vi "Modbus Message Loop.vi"(0 "Message Queues in":T1, 1 "PLC IP address":string="10.2.0.11", 3 "error in (no error)":errorcluster) -> (10 "error out":errorcluster)   [LabVIEW 2020, in "Modbus.lvlib"]
uses:
  Modbus.lvlib
  support/Message Queue/All Message Queues.ctl
  support/Message Queue/Message Cluster.ctl
  <vilib>/NI/Modbus Library/API/Master/Modbus Master.lvclass
  support/Message Queue/Enqueue Message (Single).vi
  <vilib>/NI/Modbus Library/API/Wrapper/Create TCP Master.vi
  support/Message Queue/Message Queue.lvlib
  <vilib>/NI/Modbus Library/API/Wrapper/API Main.lvlib
panel:
  out "LDO Array 2":bool[](array[boolean])
  in  "Read States":bool
  out "States":string[](array[string])
  out "TimeoutRequestGetDataLDO":u16[](array[numeric])
  out "LDO Array 1":bool[](array[boolean])
  out "Loop Count":i32
  out "FV Output":bool[](array[boolean])
  out "TimeoutRequestGetDataFVIR":i32[](array[numeric])
  out "Input Registers":u16[](array[numeric])
  # "Anybus: 192.168.0.50\nPLC: 192.168.0.20\n\nThis is available in the front HMI, e. IP and port. Useful for debugging and IP config change"
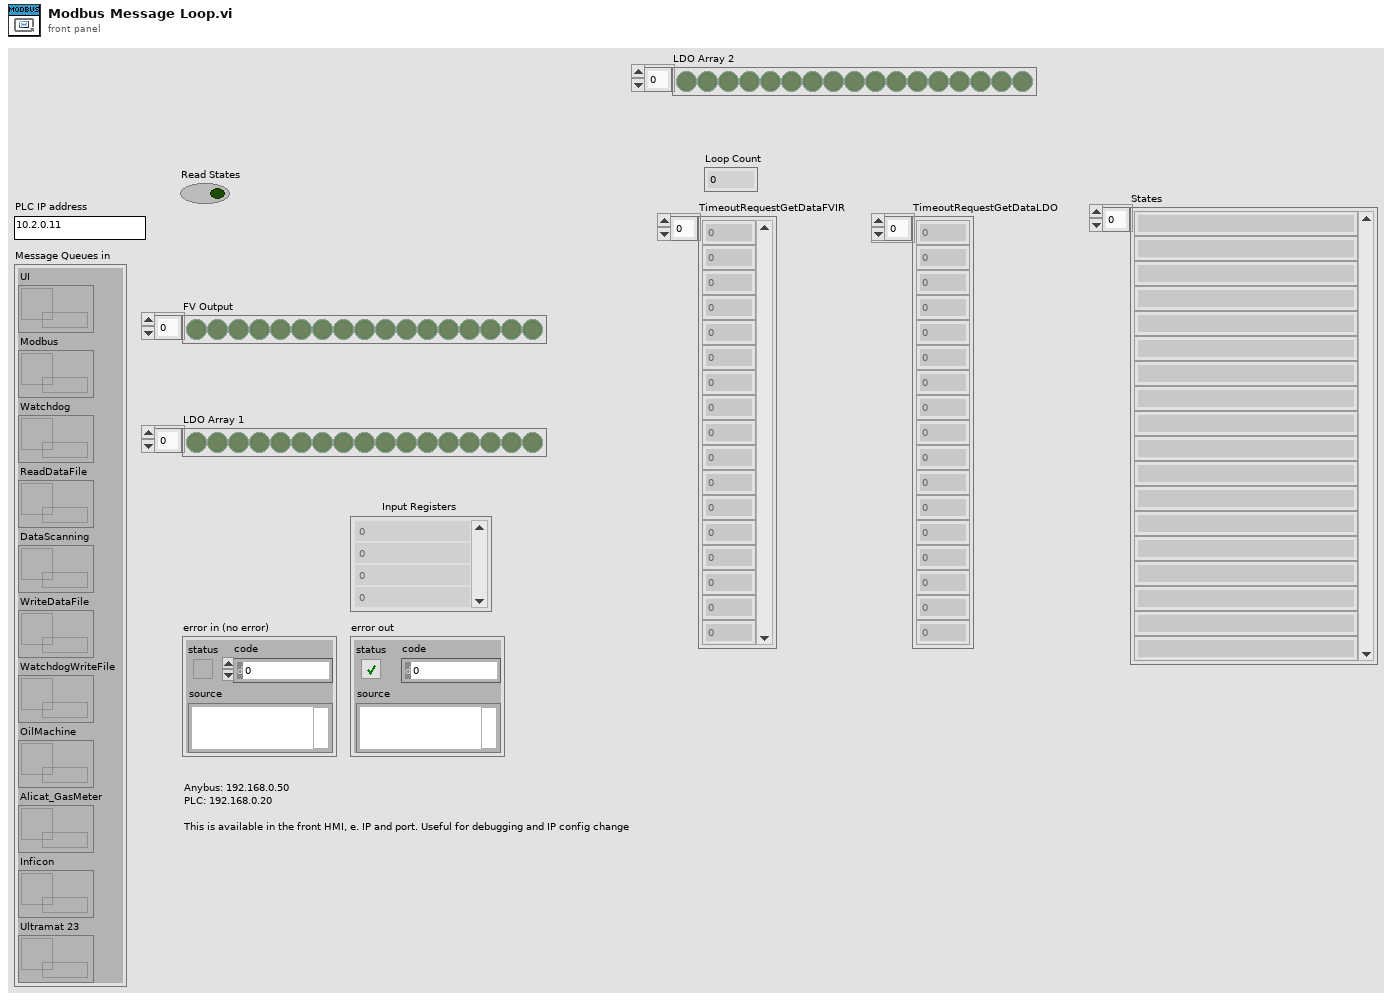
[diagram p1: front panel]
types:
  T1 = typedef "Message Queue.lvlib/All Message Queues.ctl" = cluster{"UI":refnum<queue>, "Modbus":refnum<queue>, "Watchdog":refnum<queue>, "ReadDataFile":refnum<queue>, "DataScanning":refnum<queue>, "WriteDataFile":refnum<queue>, "WatchdogWriteFile":refnum<queue>, "OilMachine":refnum<queue>, "Alicat_GasMeter":refnum<queue>, "Inficon":refnum<queue>, "Ultramat 23":refnum<queue>}
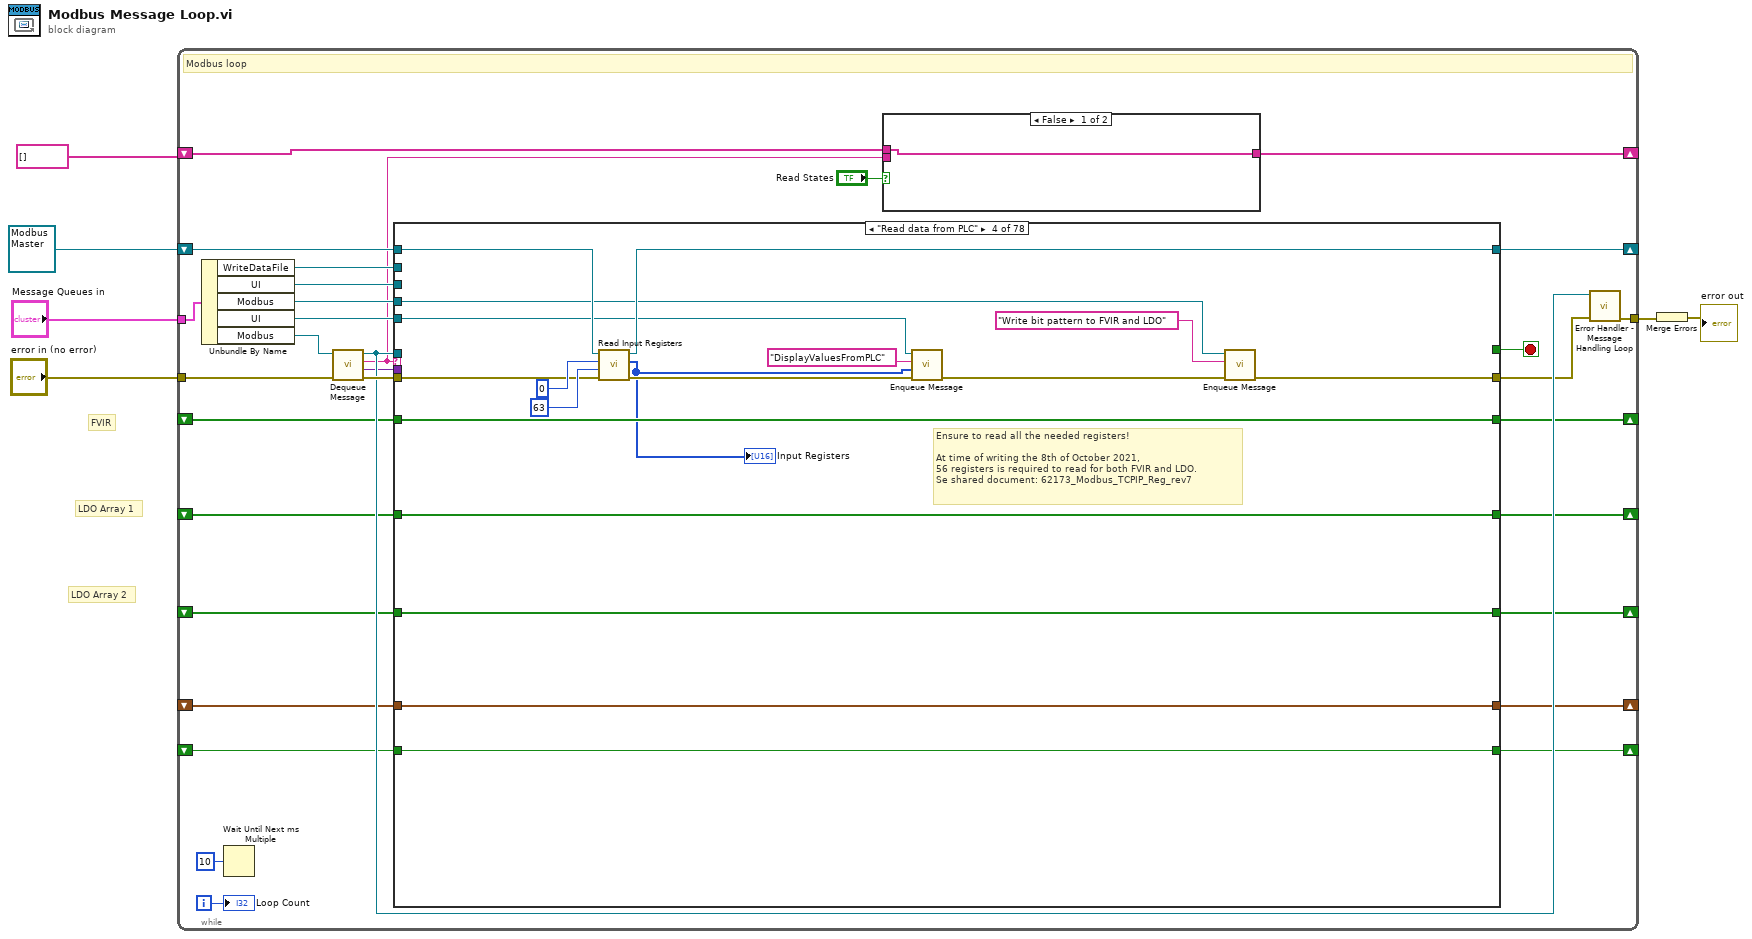
[diagram p0: block diagram]
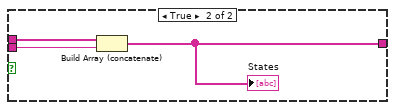
[diagram p2: hidden frame]
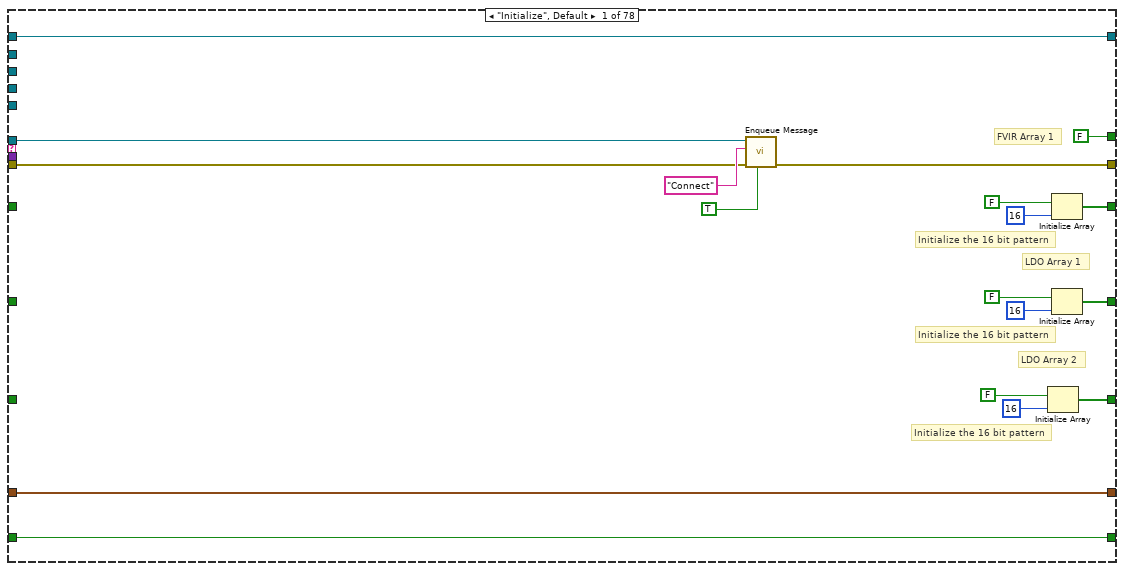
[diagram p3: hidden frame]
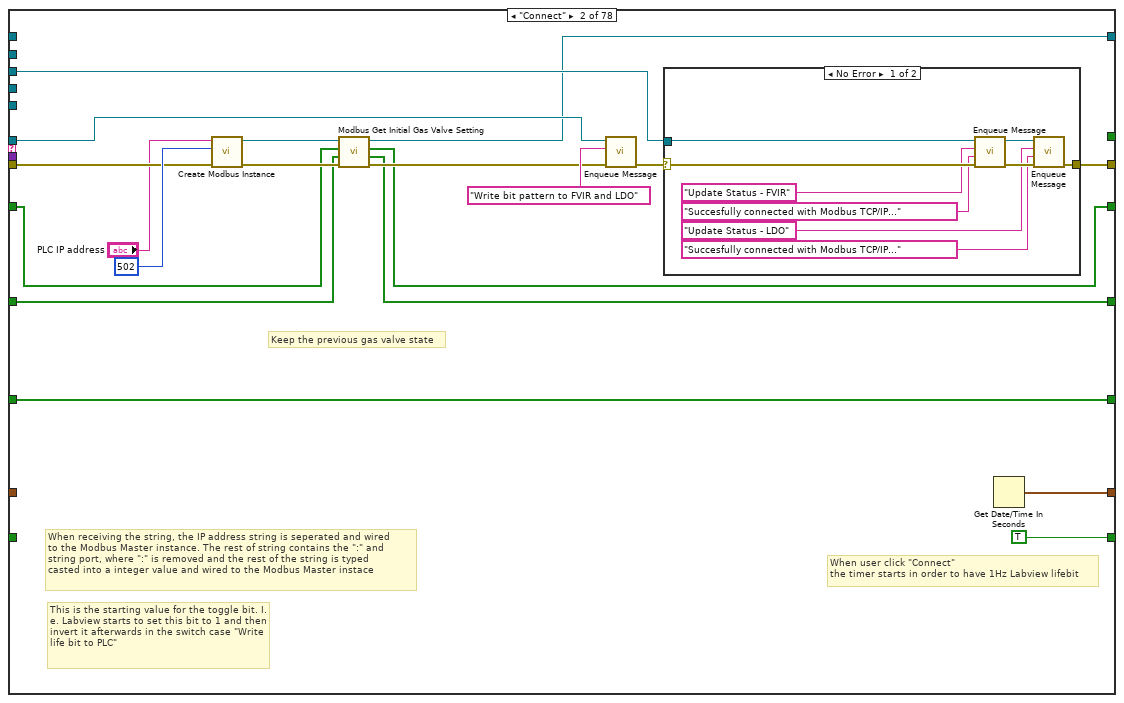
[diagram p4: hidden frame]
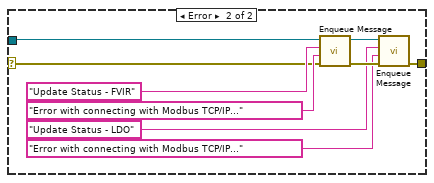
[diagram p5: hidden frame]
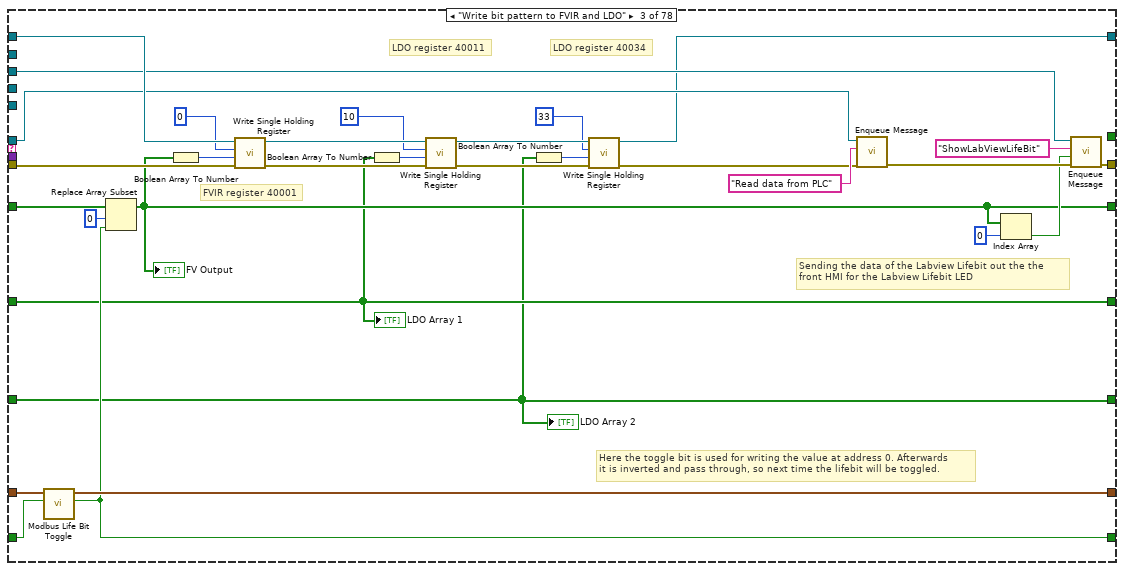
[diagram p6: hidden frame]
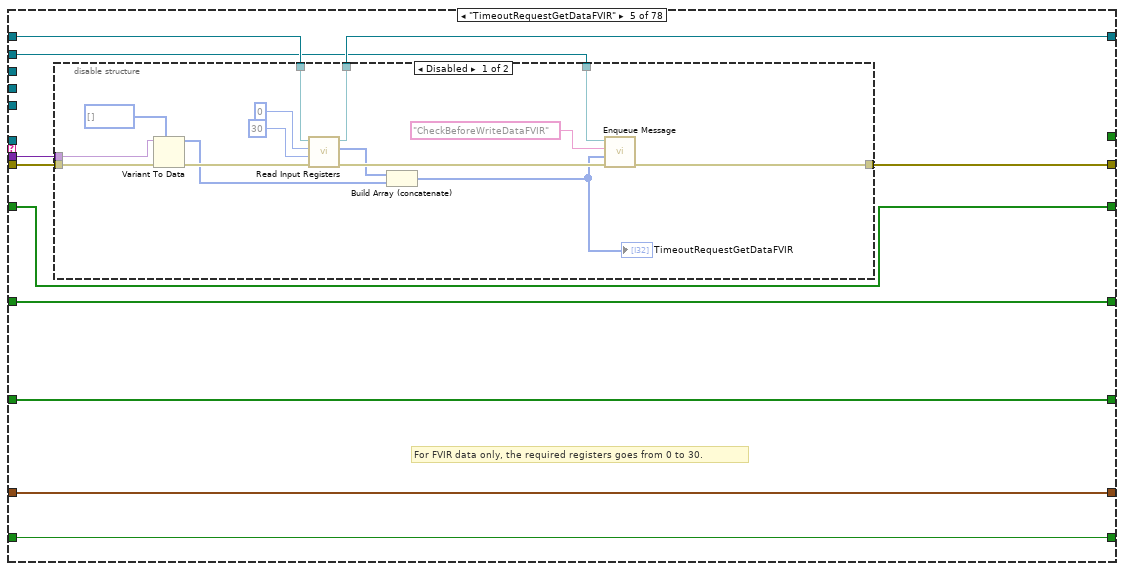
[diagram p7: hidden frame]
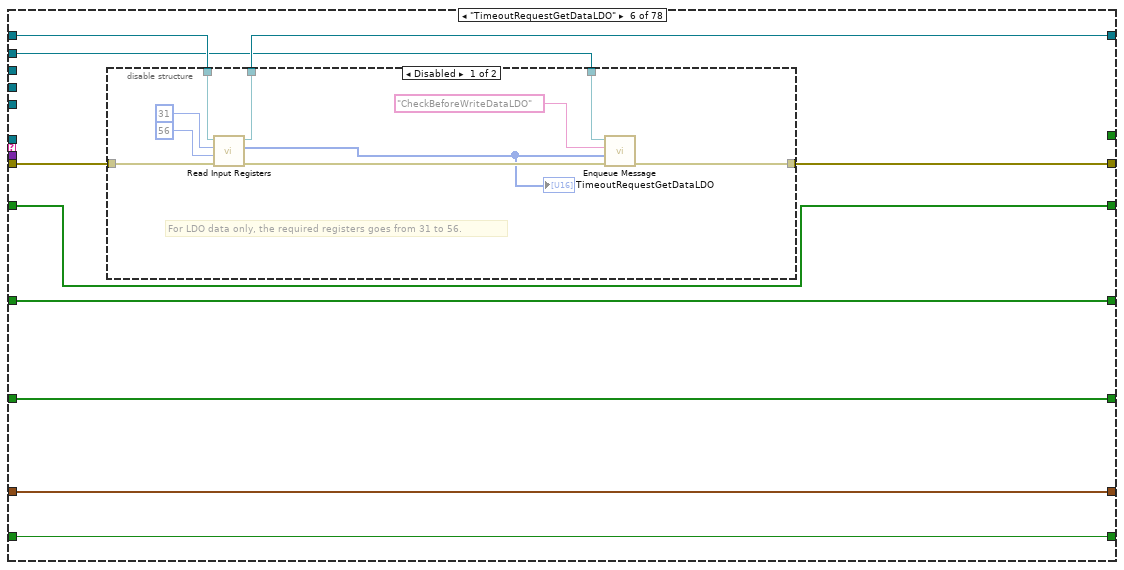
[diagram p9: hidden frame]
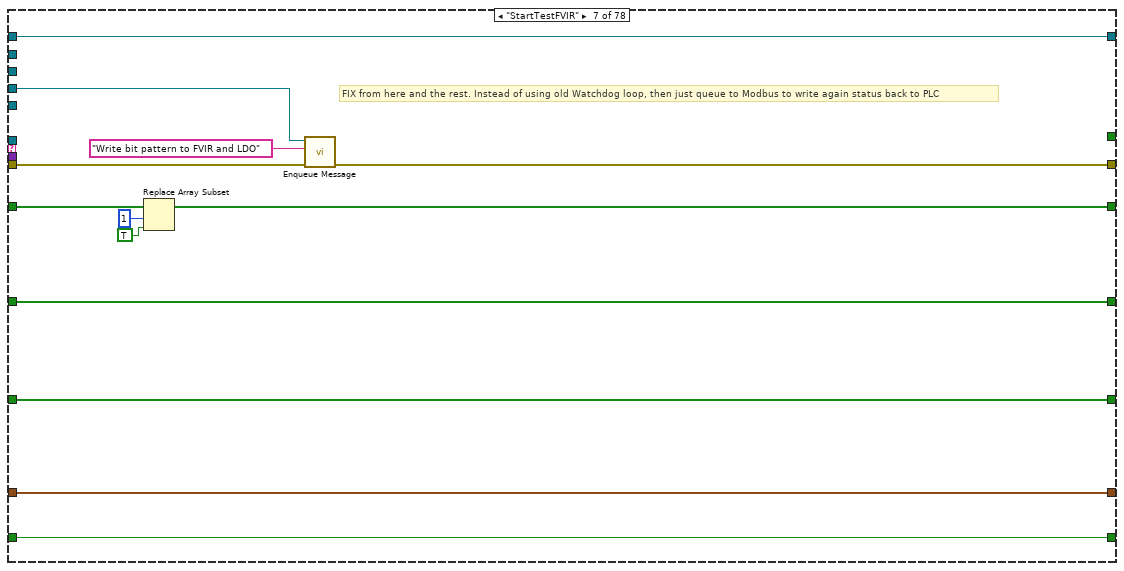
[diagram p11: hidden frame]
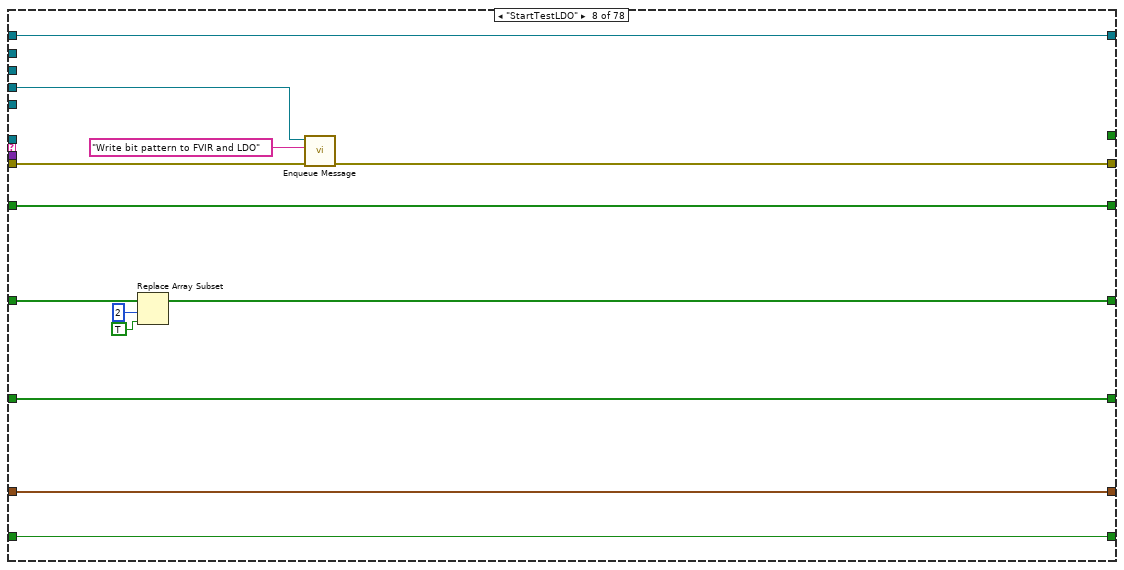
[diagram p12: hidden frame]
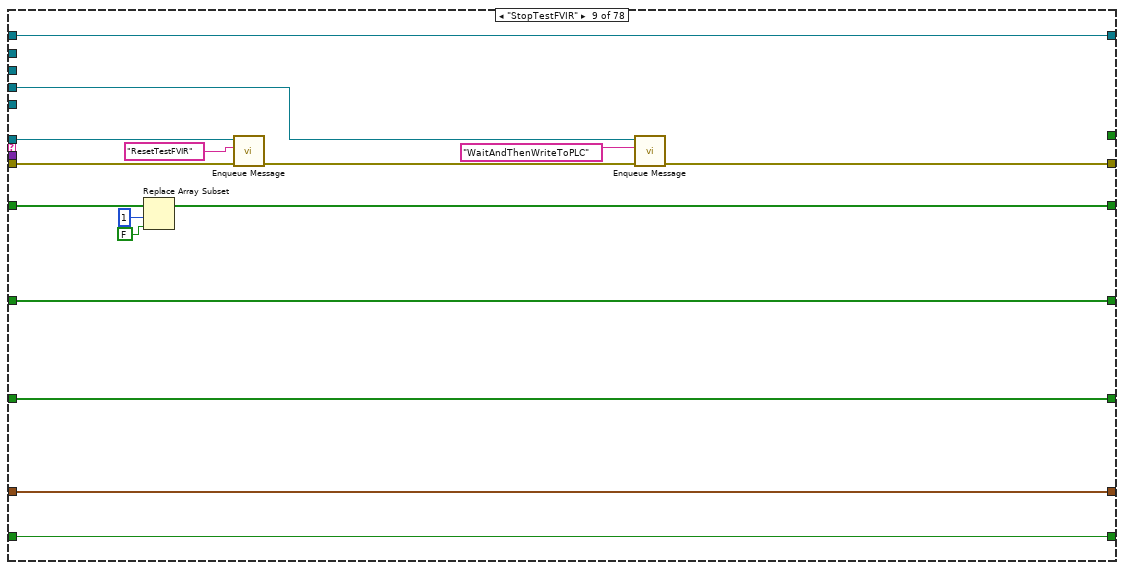
[diagram p13: hidden frame]
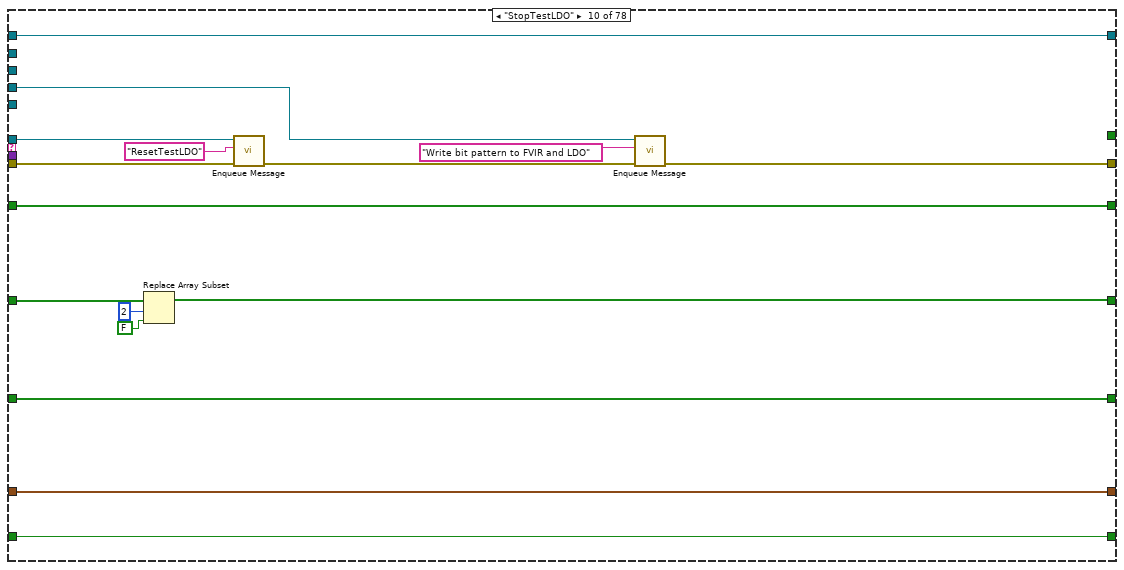
[diagram p14: hidden frame]
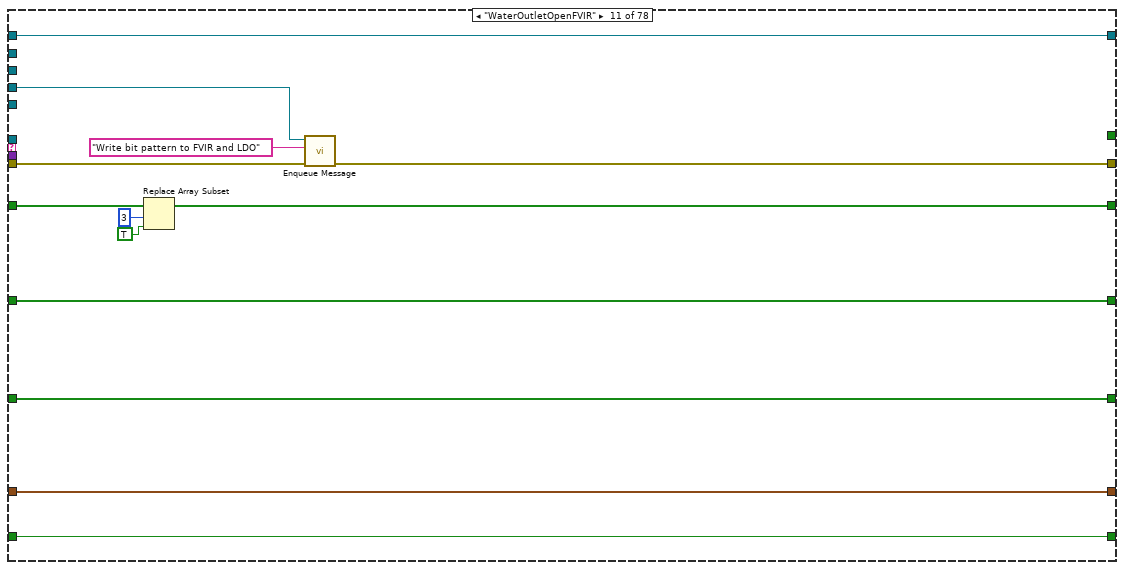
[diagram p15: hidden frame]
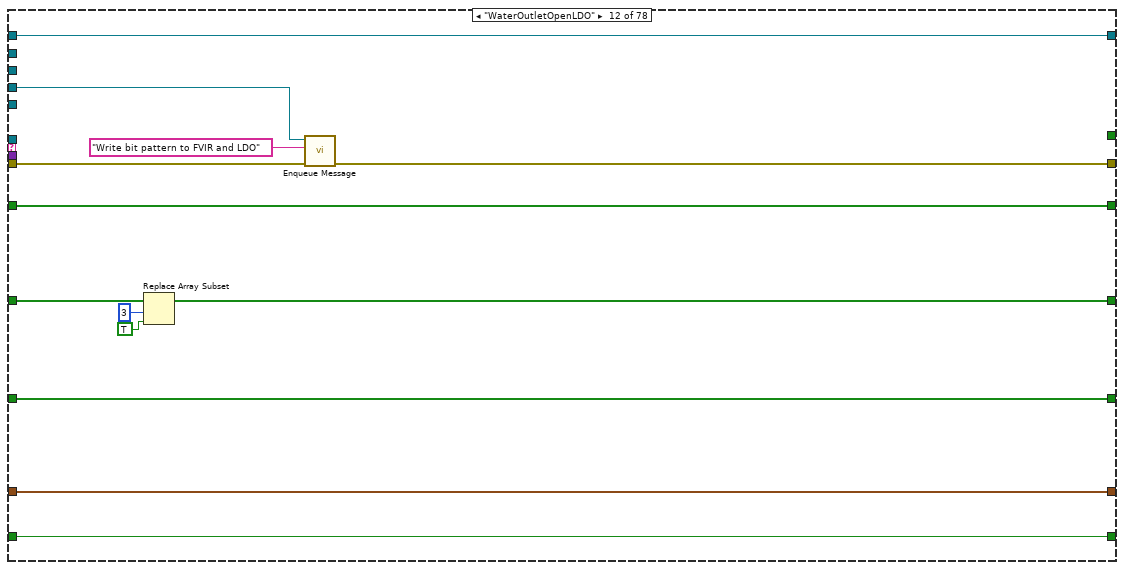
[diagram p16: hidden frame]
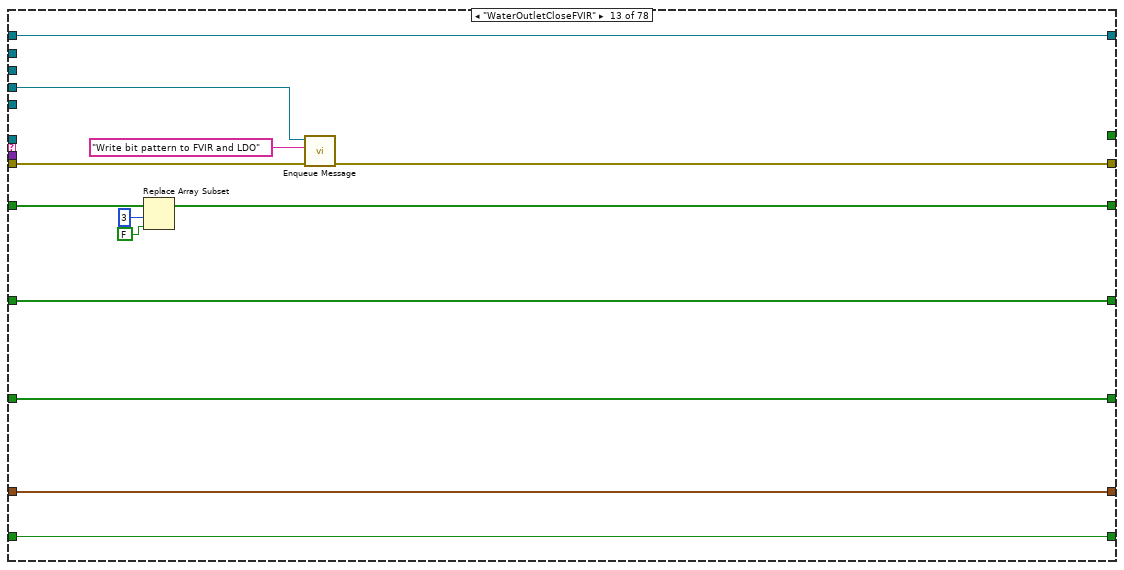
[diagram p17: hidden frame]
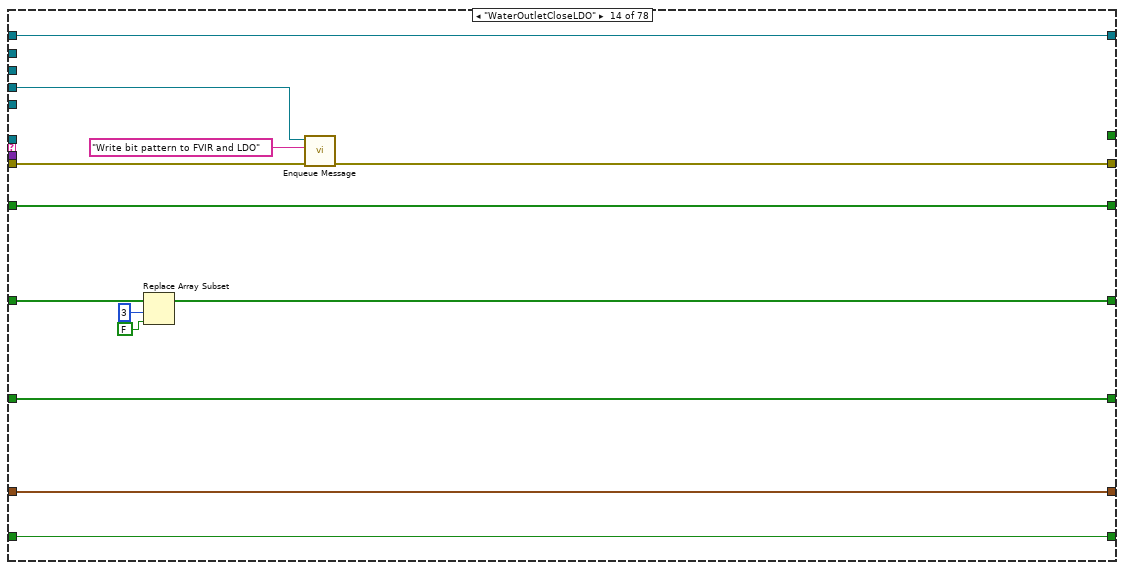
[diagram p18: hidden frame]
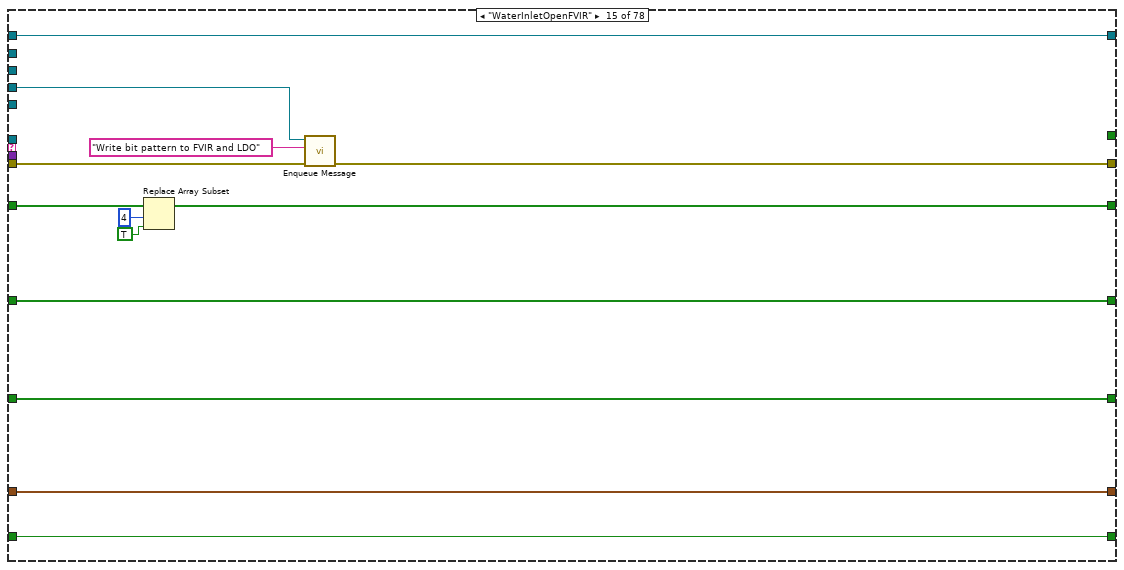
[diagram p19: hidden frame]
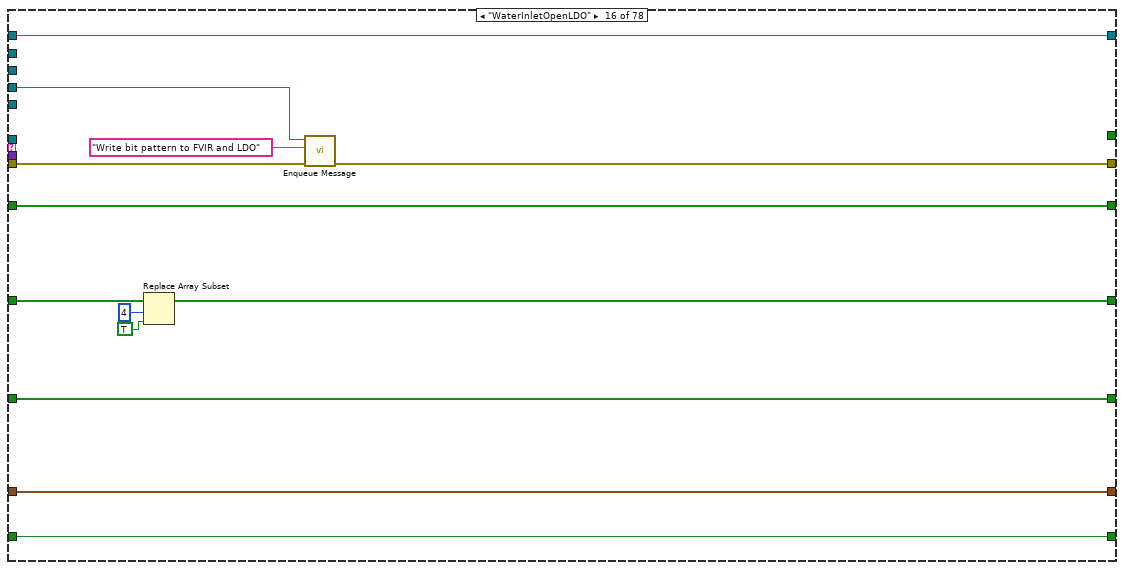
[diagram p20: hidden frame]
diagram:
  # "LDO Array 2"
  # "LDO Array 1"
  # "FVIR"
  n1 = while {
    tunnel: "Message Queues in" -> [w35]
    tunnel: [w34] -> w3
    tunnel: "error in (no error)" -> [w33]
    shift-right: [w31] -> _
    shift-left: refnum<class "Modbus Master.lvclass"> refnum ("Modbus Master") -> [w32]
    shift-right: [w25] -> _
    shift-left: _ -> [w24]
    shift-right: [w21] -> _
    shift-left: _ -> [w20]
    shift-right: [w18] -> _
    shift-left: _ -> [w17]
    shift-right: [w16] -> _
    shift-left: _ -> [w15]
    shift-right: [w10] -> _
    shift-left: string[] [] -> [w12]
    shift-right: [w8] -> _
    shift-left: _ -> [w7]
    i -> [w13]
    stop <- w36 stop-if-true
    # "Modbus loop"
    n2 = Unbundle By Name(w35) -> ("WriteDataFile"=w19:refnum<queue>, "UI"=w23:refnum<queue>, "Modbus"=w29:refnum<queue>, "UI"=w27:refnum<queue>, "Modbus"=w28:refnum<queue>)
    n3 = Wait Until Next ms Multiple(millisecond multiple=u32 10) -> ()  [unwired: 1 out]
    n4 = call "Dequeue Message.vi"("error in (no error)"=w33, "Message Queue"=w28) -> ("error out"=w37:errorcluster, "Message Data"=w26:variant, "Message"=w11:string, "dup Message Queue"=w30:refnum<queue>)  [unwired: 6 in]
    n5 = case shown="\"Read data from PLC\"" w11 {
      tunnel: w30 -> [w46 w74 w113 _ _ _ _ _ w228 w246 _ _ _ _ _ _ _ _ _ _ _ _ _ _ _ _ _ _ _ _ _ _ _ _ _ _ _ _ _ _ _ _ _ _ _ _ _ _ _ _ _ _ _ _ _ _ _ _ _ _ _ _ _ _ _ _ _ _ _ _ _ _ w1127 _ _ _ _ _]
      tunnel: w37 -> [w48 w70 w114 w137 w150 w180 w205 w217 w227 w245 w262 w275 w288 w301 w314 w327 w340 w353 w366 w379 w392 w405 w418 w431 w444 w457 w470 w483 w496 w509 w518 w529 w548 w561 w574 w587 w600 w613 w626 w639 w647 w660 w673 w686 w699 w712 w734 w745 w762 w773 w790 w801 w818 w829 w847 w861 w875 w889 w903 w917 w923 w945 w959 w973 w978 w990 w1004 w1017 _ _ w1076 w1088 w1117 w1159 w1178 w1197 w1211 w1230]
      tunnel: [w47 w77 w123 w132 w152 w178 w207 w220 w230 w248 w265 w278 w291 w304 w317 w330 w343 w356 w369 w382 w395 w408 w421 w434 w447 w460 w473 w486 w499 w512 w515 w528 w551 w564 w577 w590 w603 w616 w629 w642 w646 w659 w672 w685 w698 w711 w728 w748 w756 w776 w784 w804 w812 w832 w839 w853 w867 w881 w895 w909 w924 w937 w951 w965 w979 w992 w1005 w1018 w1037 w1061 w1072 w1081 w1110 w1148 w1166 w1185 w1205 w1224] -> w22
      tunnel: [FALSE _ _ _ _ _ _ _ _ _ _ _ _ _ _ _ _ _ _ _ _ _ _ _ _ _ _ _ _ _ _ _ _ _ _ _ _ _ _ _ _ _ _ _ _ _ _ _ _ _ _ _ _ _ _ _ _ _ _ _ _ _ _ _ _ _ _ _ _ _ _ _ TRUE _ _ _ _ _] -> w36
      tunnel: w32 -> [w59 _ w127 w144 w156 w183 w206 w218 w236 w252 w263 w276 w289 w302 w315 w328 w341 w354 w367 w380 w393 w406 w419 w432 w445 w458 w471 w484 w497 w510 w523 w536 w549 w562 w575 w588 w601 w614 w627 w640 w645 w658 w671 w684 w697 w710 w735 w746 w763 w774 w791 w802 w819 w830 w845 w859 w873 w887 w901 w915 w930 w943 w957 w971 w974 w987 w1000 w1013 w1034 w1059 w1074 w1087 w1113 w1152 w1171 w1190 w1209 w1228]
      tunnel: [w59 w65 w100 w142 w155 w182 w206 w218 w236 w252 w263 w276 w289 w302 w315 w328 w341 w354 w367 w380 w393 w406 w419 w432 w445 w458 w471 w484 w497 w510 w523 w536 w549 w562 w575 w588 w601 w614 w627 w640 w645 w658 w671 w684 w697 w710 w735 w746 w763 w774 w791 w802 w819 w830 w846 w860 w874 w888 w902 w916 w931 w944 w958 w972 w974 w987 w1000 w1013 w1033 w1058 w1075 w1087 w1113 w1151 w1170 w1189 w1208 w1227] -> w31
      tunnel: w29 -> [_ _ _ w131 _ _ w208 w221 w231 w249 w266 w279 w292 w305 w318 w331 w344 w357 w370 w383 w396 w409 w422 w435 w448 w461 w474 w487 w500 w513 w519 w530 w552 w565 w578 w591 w604 w617 w630 w643 w648 w661 w674 w687 w700 w713 w727 w749 w755 w777 w783 w805 w811 w833 w842 w856 w870 w884 w898 w912 w927 w940 w954 w968 w977 w991 w1003 w1016 w1041 w1065 _ w1085 w1116 w1147 w1168 w1187 w1204 w1223]
      tunnel: w27 -> [_ _ _ w140 _ _ _ _ _ _ _ _ _ _ _ _ _ _ _ _ _ _ _ _ _ _ _ _ _ _ _ _ _ _ _ _ _ _ _ _ _ _ _ _ _ _ _ _ _ _ _ _ _ _ _ _ _ _ _ _ _ _ _ _ _ _ _ _ _ _ _ _ w1109 _ _ _ _ _]
      tunnel: w26 -> [_ _ _ _ w149 _ _ _ _ _ _ _ _ _ _ _ _ _ _ _ _ _ _ _ _ _ _ _ _ _ _ _ _ _ _ _ _ _ _ _ _ _ _ _ _ _ _ _ _ _ _ _ _ _ _ _ _ _ _ _ _ _ _ _ _ _ _ _ w1039 w1063 _ _ _ w1158 w1177 w1196 w1210 w1229]
      tunnel: [w55 w63 w107 w138 w154 w181 w202 w212 w233 w243 w259 w270 w285 w296 w311 w322 w337 w348 w363 w374 w389 w400 w415 w426 w441 w452 w467 w478 w493 w504 w526 w539 w543 w556 w569 w582 w595 w608 w621 w634 w656 w669 w682 w695 w708 w721 w731 w742 w759 w770 w787 w798 w815 w826 w838 w852 w866 w880 w894 w908 w922 w936 w950 w964 w986 w999 w1012 w1025 w1030 w1055 w1070 w1084 w1122 w1164 w1183 w1202 w1221 w1240] -> w25
      tunnel: w24 -> [_ w64 w108 w138 w154 w181 w203 w212 w234 w243 w260 w270 w286 w296 w312 w322 w338 w348 w364 w374 w390 w400 w416 w426 w442 w452 w468 w478 w494 w504 w526 w539 w543 w556 w569 w582 w595 w608 w621 w634 w656 w669 w682 w695 w708 w721 w732 w743 w760 w771 w788 w799 w816 w827 w838 w852 w866 w880 w894 w908 w922 w936 w950 w964 w986 w999 w1012 w1025 w1030 w1055 w1070 w1084 w1122 w1164 w1183 w1202 w1221 w1240]
      tunnel: w23 -> [_ w78 w121 _ _ _ _ _ _ _ _ _ _ _ _ _ _ _ _ _ _ _ _ _ _ _ _ _ _ _ _ _ _ _ _ _ _ _ _ _ _ _ _ _ _ _ _ _ _ _ _ _ _ _ _ _ _ _ _ _ _ _ _ _ _ _ _ _ _ _ _ w1080 _ _ _ _ _ _]
      tunnel: [w52 w61 w104 w134 w153 w179 w200 w213 w225 w241 w257 w271 w283 w297 w309 w323 w335 w349 w361 w375 w387 w401 w413 w427 w439 w453 w465 w479 w491 w505 w516 w531 w544 w557 w570 w583 w596 w609 w622 w635 w650 w663 w676 w689 w702 w715 w725 w740 w753 w768 w781 w796 w809 w824 w837 w851 w865 w879 w893 w907 w921 w935 w949 w963 w985 w998 w1011 w1024 w1029 w1054 w1069 w1083 w1121 w1163 w1182 w1201 w1220 w1239] -> w21
      tunnel: w20 -> [_ w62 w104 w134 w153 w179 w200 w214 w225 w242 w257 w272 w283 w298 w309 w324 w335 w350 w361 w376 w387 w402 w413 w428 w439 w454 w465 w480 w491 w506 w517 w532 w545 w558 w571 w584 w597 w610 w623 w636 w651 w664 w677 w690 w703 w716 w725 w740 w753 w768 w781 w796 w809 w824 w837 w851 w865 w879 w893 w907 w921 w935 w949 w963 w985 w998 w1011 w1024 w1029 w1054 w1069 w1083 w1121 w1163 w1182 w1201 w1220 w1239]
      tunnel: w19 -> [_ _ _ _ w151 w177 _ _ _ _ _ _ _ _ _ _ _ _ _ _ _ _ _ _ _ _ _ _ _ _ _ _ _ _ _ _ _ _ _ _ _ _ _ _ _ _ _ _ _ _ _ _ _ _ _ _ _ _ _ _ _ _ _ _ _ _ _ _ _ _ _ _ _ _ _ _ _ _]
      tunnel: [w51 w73 w111 w130 w148 w176 w198 w211 w224 w240 w256 w269 w282 w295 w308 w321 w334 w347 w360 w373 w386 w399 w412 w425 w438 w451 w464 w477 w490 w503 w525 w538 w542 w555 w568 w581 w594 w607 w620 w633 w655 w668 w681 w694 w707 w720 w724 w739 w752 w767 w780 w795 w808 w823 w836 w850 w864 w878 w892 w906 w920 w934 w948 w962 w984 w997 w1010 w1023 w1028 w1053 w1068 w1079 w1120 w1162 w1181 w1200 w1219 w1238] -> w18
      tunnel: w17 -> [w51 _ w110 w130 w148 w176 w198 w211 w224 w240 w256 w269 w282 w295 w308 w321 w334 w347 w360 w373 w386 w399 w412 w425 w438 w451 w464 w477 w490 w503 w525 w538 w542 w555 w568 w581 w594 w607 w620 w633 w655 w668 w681 w694 w707 w720 w724 w739 w752 w767 w780 w795 w808 w823 w836 w850 w864 w878 w892 w906 w920 w934 w948 w962 w984 w997 w1010 w1023 w1028 w1053 w1068 w1079 w1120 w1162 w1181 w1200 w1219 w1238]
      tunnel: [w50 TRUE w105 w129 w147 w175 w197 w210 w223 w239 w255 w268 w281 w294 w307 w320 w333 w346 w359 w372 w385 w398 w411 w424 w437 w450 w463 w476 w489 w502 w524 w537 w541 w554 w567 w580 w593 w606 w619 w632 w654 w667 w680 w693 w706 w719 w723 w738 w751 w766 w779 w794 w807 w822 w835 w849 w863 w877 w891 w905 w919 w933 w947 w961 w983 w996 w1009 w1022 w1027 w1052 w1067 w1078 w1119 w1161 w1180 w1199 w1218 w1237] -> w16
      tunnel: w15 -> [w50 _ w109 w129 w147 w175 w197 w210 w223 w239 w255 w268 w281 w294 w307 w320 w333 w346 w359 w372 w385 w398 w411 w424 w437 w450 w463 w476 w489 w502 w524 w537 w541 w554 w567 w580 w593 w606 w619 w632 w654 w667 w680 w693 w706 w719 w723 w738 w751 w766 w779 w794 w807 w822 w835 w849 w863 w877 w891 w905 w919 w933 w947 w961 w983 w996 w1009 w1022 w1027 w1052 w1067 w1078 w1119 w1161 w1180 w1199 w1218 w1237]
      tunnel: [w43 w60 w97 w128 w146 w174 w196 w209 w222 w238 w254 w267 w280 w293 w306 w319 w332 w345 w358 w371 w384 w397 w410 w423 w436 w449 w462 w475 w488 w501 w514 w527 w540 w553 w566 w579 w592 w605 w618 w631 w644 w657 w670 w683 w696 w709 w722 w737 w750 w765 w778 w793 w806 w821 w834 w848 w862 w876 w890 w904 w918 w932 w946 w960 w975 w989 w1001 w1014 w1026 w1051 w1066 w1077 w1108 w1146 w1165 w1184 w1203 w1222] -> w8
      tunnel: w7 -> [_ w60 w97 w128 w146 w174 w196 w209 w222 w238 w254 w267 w280 w293 w306 w319 w332 w345 w358 w371 w384 w397 w410 w423 w436 w449 w462 w475 w488 w501 w514 w527 w540 w553 w566 w579 w592 w605 w618 w631 w644 w657 w670 w683 w696 w709 w722 w737 w750 w765 w778 w793 w806 w821 w834 w848 w862 w876 w890 w904 w918 w932 w946 w960 w976 w988 w1002 w1015 w1026 w1051 w1066 w1077 w1108 w1146 w1165 w1184 w1203 w1222]
      frame "Initialize", Default {
        # "LDO Array 2"
        # "Initialize the 16 bit pattern"
        # "LDO Array 1"
        # "FVIR Array 1"
        # "Initialize the 16 bit pattern"
        # "Initialize the 16 bit pattern"
        n6 = call-poly "Enqueue Message.vi"("Priority Message? (F)"=TRUE, "error in (no error)"=w48, "Message"="Connect", "Message Queue"=w46) -> ("error out"=w47:errorcluster)  [unwired: 6 in, 1 out]
        n7 = Initialize Array(FALSE, 16 ("dimension size")) -> (w43:bool[])
        n8 = Initialize Array(FALSE, 16 ("dimension size")) -> (w55:bool[])
        n9 = Initialize Array(FALSE, 16 ("dimension size")) -> (w52:bool[])
      }
      frame "Connect" {
        # "Keep the previous gas valve state"
        # "When user click \"Connect\"\nthe timer starts in order to have 1Hz Labview lifebit"
        # "When receiving the string, the IP address string is seperated and wired\nto the Modbus Master instance. The rest of string contains the \":\" and\nstring port, where \":\" is removed and the rest of the string is typed \ncasted into a integer value and wired to the Modbus Master instace"
        # "This is the starting value for the toggle bit. I.e. Labview starts to set this bit to 1 and then invert it afterwards in the switch case \"Write life bit to PLC\""
        n10 = call-poly <vilib>:"Create Modbus Instance.vi"("error in"=w70, "port (502)"=u16 502 ("Port"), "address"="PLC IP address") -> ("error out"=w68:errorcluster, "TCP master instance"=w66:refnum<class "Modbus Master.lvclass">)  [unwired: 7 in]
        n11 = call "Modbus Get Initial Gas Valve Setting.vi"("error in (no error)"=w68, "LDO Input"=w62, "FVIR Input"=w64, "Modbus Master in"=w66) -> ("error out"=w67:errorcluster, "LDO Output"=w61:bool[], "FVIR Output"=w63:bool[], "Modbus Master out"=w65:refnum<class "Modbus Master.lvclass">)  [unwired: 4 in]
        n12 = call-poly "Enqueue Message.vi"("error in (no error)"=w67, "Message"="Write bit pattern to FVIR and LDO", "Message Queue"=w74) -> ("error out"=w75:errorcluster)  [unwired: 7 in, 1 out]
        n13 = case shown="No Error" w75 {
          selector: w75 -> [w87 w90]
          tunnel: w78 -> [w79 w88]
          tunnel: [w85 w89] -> w77
          frame No Error {
            n14 = call-poly "Enqueue Message.vi"("error in (no error)"=w87, "Message Data"="Succesfully connected with Modbus TCP/IP..." ("Acquiring and Logging..."), "Message"="Update Status - FVIR", "Message Queue"=w79) -> ("error out"=w86:errorcluster, "dup Message Queue"=w84:refnum<queue>)  [unwired: 6 in]
            n15 = call-poly "Enqueue Message.vi"("error in (no error)"=w86, "Message Data"="Succesfully connected with Modbus TCP/IP..." ("Acquiring and Logging..."), "Message"="Update Status - LDO", "Message Queue"=w84) -> ("error out"=w85:errorcluster)  [unwired: 6 in, 1 out]
          }
          frame Error {
            n16 = call-poly "Enqueue Message.vi"("error in (no error)"=w90, "Message Data"="Error with connecting with Modbus TCP/IP..." ("Acquiring and Logging..."), "Message"="Update Status - FVIR", "Message Queue"=w88) -> ("error out"=w96:errorcluster, "dup Message Queue"=w95:refnum<queue>)  [unwired: 6 in]
            n17 = call-poly "Enqueue Message.vi"("error in (no error)"=w96, "Message Data"="Error with connecting with Modbus TCP/IP..." ("Acquiring and Logging..."), "Message"="Update Status - LDO", "Message Queue"=w95) -> ("error out"=w89:errorcluster)  [unwired: 6 in, 1 out]
          }
        }
        n18 = Get Date/Time In Seconds() -> (seconds since 1Jan1904=w73:timestamp)
      }
      frame "Write bit pattern to FVIR and LDO" {
        # "LDO register 40034"
        # "LDO register 40011"
        # "FVIR register 40001"
        # "Sending the data of the Labview Lifebit out the the \nfront HMI for the Labview Lifebit LED"
        # "Here the toggle bit is used for writing the value at address 0. Afterwards\nit is inverted and pass through, so next time the lifebit will be toggled."
        n19 = call "Modbus Life Bit Toggle.vi"("Toggle Input"=w109, "seconds since 1Jan1904 in"=w110) -> ("Toggle Output"=w105:bool, "seconds since 1Jan1904 out"=w111:timestamp)  [unwired: 8 in]
        n20 = Replace Array Subset(array=w108, new element=w105, index=0) -> (w107:bool[])
        "FV Output" <- w107
        n21 = Boolean Array To Number(Boolean array=w107) -> (number=w125:u32)
        n22 = call-dynamic "Write Single Holding Register.vi"("error in"=w114, "register to write"=w125, "address"=u16 0 ("starting address"), "Modbus master in"=w127) -> ("error out"=w117:errorcluster, "Modbus master out"=w118:refnum<class "Modbus Master.lvclass">)  [unwired: 6 in]
        n23 = Boolean Array To Number(Boolean array=w104) -> (number=w115:u32)
        n24 = call-dynamic "Write Single Holding Register.vi"("error in"=w117, "register to write"=w115, "address"=u16 10, "Modbus master in"=w118) -> ("error out"=w103:errorcluster, "Modbus master out"=w101:refnum<class "Modbus Master.lvclass">)  [unwired: 6 in]
        n25 = Boolean Array To Number(Boolean array=w97) -> (number=w98:u32)
        n26 = call-dynamic "Write Single Holding Register.vi"("error in"=w103, "register to write"=w98, "address"=u16 33, "Modbus master in"=w101) -> ("error out"=w102:errorcluster, "Modbus master out"=w100:refnum<class "Modbus Master.lvclass">)  [unwired: 6 in]
        n27 = call-poly "Enqueue Message.vi"("error in (no error)"=w102, "Message"="Read data from PLC", "Message Queue"=w113) -> ("error out"=w124:errorcluster)  [unwired: 7 in, 1 out]
        n28 = Index Array(array=w107, index=0) -> (element=w119:bool)
        n29 = call-poly "Enqueue Message.vi"("error in (no error)"=w124, "Message Data"=w119, "Message"="ShowLabViewLifeBit", "Message Queue"=w121) -> ("error out"=w123:errorcluster)  [unwired: 6 in, 1 out]
        "LDO Array 1" <- w104
        "LDO Array 2" <- w97
      }
      frame "Read data from PLC" {
        # "Ensure to read all the needed registers! \n\nAt time of writing the 8th of October 2021, \n56 registers is required to read for both FVIR and LDO. \nSe shared document: 62173_Modbus_TCPIP_Reg_rev7"
        n30 = call-dynamic "Read Input Registers.vi"("error in"=w137, "number of inputs"=u16 63, "starting address"=u16 0, "Modbus master in"=w144) -> ("error out"=w136:errorcluster, "register values"=w133:u16[], "Modbus master out"=w142:refnum<class "Modbus Master.lvclass">)  [unwired: 5 in]
        "Input Registers" <- w133
        n31 = call-poly "Enqueue Message.vi"("error in (no error)"=w136, "Message Data"=w133, "Message"="DisplayValuesFromPLC", "Message Queue"=w140) -> ("error out"=w135:errorcluster)  [unwired: 6 in, 1 out]
        n32 = call-poly "Enqueue Message.vi"("error in (no error)"=w135, "Message"="Write bit pattern to FVIR and LDO", "Message Queue"=w131) -> ("error out"=w132:errorcluster)  [unwired: 7 in, 1 out]
      }
      frame "TimeoutRequestGetDataFVIR" {
        # "For FVIR data only, the required registers goes from 0 to 30."
        n33 = disable-structure shown="Disabled" {
          disable-tunnel: w156 -> [w170 w173]
          disable-tunnel: [w168 w173] -> w155
          disable-tunnel: [w166 w172] -> w152
          disable-tunnel: w151 -> [w165 _]
          disable-tunnel: w150 -> [w163 w172]
          disable-tunnel: w149 -> [w160 _]
          frame Disabled {
            n34 = Variant To Data(error in=w163, type=i32[] [], Variant=w160) -> (data=w158:i32[], error out=w162:errorcluster)
            n35 = call-dynamic "Read Input Registers.vi"("error in"=w162, "number of inputs"=u16 30, "starting address"=u16 0, "Modbus master in"=w170) -> ("error out"=w167:errorcluster, "register values"=w159:u16[], "Modbus master out"=w168:refnum<class "Modbus Master.lvclass">)  [unwired: 5 in]
            n36 = Build Array (concatenate)(w159, w158) -> (w157:i32[])
            "TimeoutRequestGetDataFVIR" <- w157
            n37 = call-poly "Enqueue Message.vi"("error in (no error)"=w167, "Message Data"=w157, "Message"="CheckBeforeWriteDataFVIR", "Message Queue"=w165) -> ("error out"=w166:errorcluster)  [unwired: 6 in, 1 out]
          }
          frame Enabled {
          }
        }
      }
      frame "TimeoutRequestGetDataLDO" {
        n38 = disable-structure shown="Disabled" {
          disable-tunnel: w183 -> [w192 w194]
          disable-tunnel: [w190 w194] -> w182
          disable-tunnel: w180 -> [w189 w195]
          disable-tunnel: [w187 w195] -> w178
          disable-tunnel: w177 -> [w186 _]
          frame Disabled {
            # "For LDO data only, the required registers goes from 31 to 56."
            n39 = call-dynamic "Read Input Registers.vi"("error in"=w189, "number of inputs"=u16 56, "starting address"=u16 31, "Modbus master in"=w192) -> ("error out"=w188:errorcluster, "register values"=w185:u16[], "Modbus master out"=w190:refnum<class "Modbus Master.lvclass">)  [unwired: 5 in]
            "TimeoutRequestGetDataLDO" <- w185
            n40 = call-poly "Enqueue Message.vi"("error in (no error)"=w188, "Message Data"=w185, "Message"="CheckBeforeWriteDataLDO", "Message Queue"=w186) -> ("error out"=w187:errorcluster)  [unwired: 6 in, 1 out]
          }
          frame Enabled {
          }
        }
      }
      frame "StartTestFVIR" {
        # "FIX from here and the rest. Instead of using old Watchdog loop, then just queue to Modbus to write again status back to PLC"
        n41 = Replace Array Subset(array=w203, new element=TRUE ("new element/subarray"), index=1) -> (w202:bool[])
        n42 = call-poly "Enqueue Message.vi"("error in (no error)"=w205, "Message"="Write bit pattern to FVIR and LDO", "Message Queue"=w208) -> ("error out"=w207:errorcluster)  [unwired: 7 in, 1 out]
      }
      frame "StartTestLDO" {
        n43 = Replace Array Subset(array=w214, new element=TRUE ("new element/subarray"), index=2) -> (w213:bool[])
        n44 = call-poly "Enqueue Message.vi"("error in (no error)"=w217, "Message"="Write bit pattern to FVIR and LDO", "Message Queue"=w221) -> ("error out"=w220:errorcluster)  [unwired: 7 in, 1 out]
      }
      frame "StopTestFVIR" {
        n45 = Replace Array Subset(array=w234, new element=FALSE ("new element/subarray"), index=1) -> (w233:bool[])
        n46 = call-poly "Enqueue Message.vi"("error in (no error)"=w227, "Message"="ResetTestFVIR", "Message Queue"=w228) -> ("error out"=w226:errorcluster)  [unwired: 7 in, 1 out]
        n47 = call-poly "Enqueue Message.vi"("error in (no error)"=w226, "Message"="WaitAndThenWriteToPLC", "Message Queue"=w231) -> ("error out"=w230:errorcluster)  [unwired: 7 in, 1 out]
      }
      frame "StopTestLDO" {
        n48 = Replace Array Subset(array=w242, new element=FALSE ("new element/subarray"), index=2) -> (w241:bool[])
        n49 = call-poly "Enqueue Message.vi"("error in (no error)"=w245, "Message"="ResetTestLDO", "Message Queue"=w246) -> ("error out"=w244:errorcluster)  [unwired: 7 in, 1 out]
        n50 = call-poly "Enqueue Message.vi"("error in (no error)"=w244, "Message"="Write bit pattern to FVIR and LDO", "Message Queue"=w249) -> ("error out"=w248:errorcluster)  [unwired: 7 in, 1 out]
      }
      frame "WaterOutletOpenFVIR" {
        n51 = Replace Array Subset(array=w260, new element=TRUE ("new element/subarray"), index=3) -> (w259:bool[])
        n52 = call-poly "Enqueue Message.vi"("error in (no error)"=w262, "Message"="Write bit pattern to FVIR and LDO", "Message Queue"=w266) -> ("error out"=w265:errorcluster)  [unwired: 7 in, 1 out]
      }
      frame "WaterOutletOpenLDO" {
        n53 = Replace Array Subset(array=w272, new element=TRUE ("new element/subarray"), index=3) -> (w271:bool[])
        n54 = call-poly "Enqueue Message.vi"("error in (no error)"=w275, "Message"="Write bit pattern to FVIR and LDO", "Message Queue"=w279) -> ("error out"=w278:errorcluster)  [unwired: 7 in, 1 out]
      }
      frame "WaterOutletCloseFVIR" {
        n55 = Replace Array Subset(array=w286, new element=FALSE ("new element/subarray"), index=3) -> (w285:bool[])
        n56 = call-poly "Enqueue Message.vi"("error in (no error)"=w288, "Message"="Write bit pattern to FVIR and LDO", "Message Queue"=w292) -> ("error out"=w291:errorcluster)  [unwired: 7 in, 1 out]
      }
      frame "WaterOutletCloseLDO" {
        n57 = Replace Array Subset(array=w298, new element=FALSE ("new element/subarray"), index=3) -> (w297:bool[])
        n58 = call-poly "Enqueue Message.vi"("error in (no error)"=w301, "Message"="Write bit pattern to FVIR and LDO", "Message Queue"=w305) -> ("error out"=w304:errorcluster)  [unwired: 7 in, 1 out]
      }
      frame "WaterInletOpenFVIR" {
        n59 = Replace Array Subset(array=w312, new element=TRUE ("new element/subarray"), index=4) -> (w311:bool[])
        n60 = call-poly "Enqueue Message.vi"("error in (no error)"=w314, "Message"="Write bit pattern to FVIR and LDO", "Message Queue"=w318) -> ("error out"=w317:errorcluster)  [unwired: 7 in, 1 out]
      }
      frame "WaterInletOpenLDO" {
        n61 = Replace Array Subset(array=w324, new element=TRUE ("new element/subarray"), index=4) -> (w323:bool[])
        n62 = call-poly "Enqueue Message.vi"("error in (no error)"=w327, "Message"="Write bit pattern to FVIR and LDO", "Message Queue"=w331) -> ("error out"=w330:errorcluster)  [unwired: 7 in, 1 out]
      }
      frame "WaterInletCloseFVIR" {
        n63 = Replace Array Subset(array=w338, new element=FALSE ("new element/subarray"), index=4) -> (w337:bool[])
        n64 = call-poly "Enqueue Message.vi"("error in (no error)"=w340, "Message"="Write bit pattern to FVIR and LDO", "Message Queue"=w344) -> ("error out"=w343:errorcluster)  [unwired: 7 in, 1 out]
      }
      frame "WaterInletCloseLDO" {
        n65 = Replace Array Subset(array=w350, new element=FALSE ("new element/subarray"), index=4) -> (w349:bool[])
        n66 = call-poly "Enqueue Message.vi"("error in (no error)"=w353, "Message"="Write bit pattern to FVIR and LDO", "Message Queue"=w357) -> ("error out"=w356:errorcluster)  [unwired: 7 in, 1 out]
      }
      frame "GasSolenoidOpenFVIR" {
        n67 = Replace Array Subset(array=w364, new element=TRUE ("new element/subarray"), index=5) -> (w363:bool[])
        n68 = call-poly "Enqueue Message.vi"("error in (no error)"=w366, "Message"="Write bit pattern to FVIR and LDO", "Message Queue"=w370) -> ("error out"=w369:errorcluster)  [unwired: 7 in, 1 out]
      }
      frame "GasSolenoidOpenLDO" {
        n69 = Replace Array Subset(array=w376, new element=TRUE ("new element/subarray"), index=5) -> (w375:bool[])
        n70 = call-poly "Enqueue Message.vi"("error in (no error)"=w379, "Message"="Write bit pattern to FVIR and LDO", "Message Queue"=w383) -> ("error out"=w382:errorcluster)  [unwired: 7 in, 1 out]
      }
      frame "GasSolenoidCloseFVIR" {
        n71 = Replace Array Subset(array=w390, new element=FALSE ("new element/subarray"), index=5) -> (w389:bool[])
        n72 = call-poly "Enqueue Message.vi"("error in (no error)"=w392, "Message"="Write bit pattern to FVIR and LDO", "Message Queue"=w396) -> ("error out"=w395:errorcluster)  [unwired: 7 in, 1 out]
      }
      frame "GasSolenoidCloseLDO" {
        n73 = Replace Array Subset(array=w402, new element=FALSE ("new element/subarray"), index=5) -> (w401:bool[])
        n74 = call-poly "Enqueue Message.vi"("error in (no error)"=w405, "Message"="Write bit pattern to FVIR and LDO", "Message Queue"=w409) -> ("error out"=w408:errorcluster)  [unwired: 7 in, 1 out]
      }
      frame "WaterFlowOpenFVIR" {
        n75 = Replace Array Subset(array=w416, new element=TRUE ("new element/subarray"), index=6) -> (w415:bool[])
        n76 = call-poly "Enqueue Message.vi"("error in (no error)"=w418, "Message"="Write bit pattern to FVIR and LDO", "Message Queue"=w422) -> ("error out"=w421:errorcluster)  [unwired: 7 in, 1 out]
      }
      frame "WaterFlowStartLDO" {
        n77 = Replace Array Subset(array=w428, new element=TRUE ("new element/subarray"), index=6) -> (w427:bool[])
        n78 = call-poly "Enqueue Message.vi"("error in (no error)"=w431, "Message"="Write bit pattern to FVIR and LDO", "Message Queue"=w435) -> ("error out"=w434:errorcluster)  [unwired: 7 in, 1 out]
      }
      frame "WaterFlowCloseFVIR" {
        n79 = Replace Array Subset(array=w442, new element=FALSE ("new element/subarray"), index=6) -> (w441:bool[])
        n80 = call-poly "Enqueue Message.vi"("error in (no error)"=w444, "Message"="Write bit pattern to FVIR and LDO", "Message Queue"=w448) -> ("error out"=w447:errorcluster)  [unwired: 7 in, 1 out]
      }
      frame "WaterFlowStartZeroLDO" {
        n81 = Replace Array Subset(array=w454, new element=FALSE ("new element/subarray"), index=6) -> (w453:bool[])
        n82 = call-poly "Enqueue Message.vi"("error in (no error)"=w457, "Message"="Write bit pattern to FVIR and LDO", "Message Queue"=w461) -> ("error out"=w460:errorcluster)  [unwired: 7 in, 1 out]
      }
      frame "WaterFlowPropOpenFVIR" {
        n83 = Replace Array Subset(array=w468, new element=TRUE ("new element/subarray"), index=7) -> (w467:bool[])
        n84 = call-poly "Enqueue Message.vi"("error in (no error)"=w470, "Message"="Write bit pattern to FVIR and LDO", "Message Queue"=w474) -> ("error out"=w473:errorcluster)  [unwired: 7 in, 1 out]
      }
      frame "WaterFlowPropOpenLDO" {
        # "This is not used. Remove at some point."
        n85 = Replace Array Subset(array=w480, new element=TRUE ("new element/subarray"), index=7) -> (w479:bool[])
        n86 = call-poly "Enqueue Message.vi"("error in (no error)"=w483, "Message"="Write bit pattern to FVIR and LDO", "Message Queue"=w487) -> ("error out"=w486:errorcluster)  [unwired: 7 in, 1 out]
      }
      frame "WaterFlowPropCloseFVIR" {
        n87 = Replace Array Subset(array=w494, new element=FALSE ("new element/subarray"), index=7) -> (w493:bool[])
        n88 = call-poly "Enqueue Message.vi"("error in (no error)"=w496, "Message"="Write bit pattern to FVIR and LDO", "Message Queue"=w500) -> ("error out"=w499:errorcluster)  [unwired: 7 in, 1 out]
      }
      frame "WaterFlowPropCloseLDO" {
        # "This is not used. Remove at some point."
        n89 = Replace Array Subset(array=w506, new element=FALSE ("new element/subarray"), index=7) -> (w505:bool[])
        n90 = call-poly "Enqueue Message.vi"("error in (no error)"=w509, "Message"="Write bit pattern to FVIR and LDO", "Message Queue"=w513) -> ("error out"=w512:errorcluster)  [unwired: 7 in, 1 out]
      }
      frame "WaterFlowStopLDO" {
        n91 = Replace Array Subset(array=w517, new element=TRUE ("new element/subarray"), index=8) -> (w516:bool[])
        n92 = call-poly "Enqueue Message.vi"("error in (no error)"=w518, "Message"="Write bit pattern to FVIR and LDO", "Message Queue"=w519) -> ("error out"=w515:errorcluster)  [unwired: 7 in, 1 out]
      }
      frame "WaterFlowStopZeroLDO" {
        n93 = Replace Array Subset(array=w532, new element=FALSE ("new element/subarray"), index=8) -> (w531:bool[])
        n94 = call-poly "Enqueue Message.vi"("error in (no error)"=w529, "Message"="Write bit pattern to FVIR and LDO", "Message Queue"=w530) -> ("error out"=w528:errorcluster)  [unwired: 7 in, 1 out]
      }
      frame "OilSpray08Open" {
        n95 = Replace Array Subset(array=w545, new element=TRUE ("new element/subarray"), index=9) -> (w544:bool[])
        n96 = call-poly "Enqueue Message.vi"("error in (no error)"=w548, "Message"="Write bit pattern to FVIR and LDO", "Message Queue"=w552) -> ("error out"=w551:errorcluster)  [unwired: 7 in, 1 out]
      }
      frame "OilSpray08Close" {
        n97 = Replace Array Subset(array=w558, new element=FALSE ("new element/subarray"), index=9) -> (w557:bool[])
        n98 = call-poly "Enqueue Message.vi"("error in (no error)"=w561, "Message"="Write bit pattern to FVIR and LDO", "Message Queue"=w565) -> ("error out"=w564:errorcluster)  [unwired: 7 in, 1 out]
      }
      frame "OilSpray11Open" {
        n99 = Replace Array Subset(array=w571, new element=TRUE ("new element/subarray"), index=10) -> (w570:bool[])
        n100 = call-poly "Enqueue Message.vi"("error in (no error)"=w574, "Message"="Write bit pattern to FVIR and LDO", "Message Queue"=w578) -> ("error out"=w577:errorcluster)  [unwired: 7 in, 1 out]
      }
      frame "OilSpray11Close" {
        n101 = Replace Array Subset(array=w584, new element=FALSE ("new element/subarray"), index=10) -> (w583:bool[])
        n102 = call-poly "Enqueue Message.vi"("error in (no error)"=w587, "Message"="Write bit pattern to FVIR and LDO", "Message Queue"=w591) -> ("error out"=w590:errorcluster)  [unwired: 7 in, 1 out]
      }
      frame "OilSpray133Open" {
        n103 = Replace Array Subset(array=w597, new element=TRUE ("new element/subarray"), index=11) -> (w596:bool[])
        n104 = call-poly "Enqueue Message.vi"("error in (no error)"=w600, "Message"="Write bit pattern to FVIR and LDO", "Message Queue"=w604) -> ("error out"=w603:errorcluster)  [unwired: 7 in, 1 out]
      }
      frame "OilSpray133Close" {
        n105 = Replace Array Subset(array=w610, new element=FALSE ("new element/subarray"), index=11) -> (w609:bool[])
        n106 = call-poly "Enqueue Message.vi"("error in (no error)"=w613, "Message"="Write bit pattern to FVIR and LDO", "Message Queue"=w617) -> ("error out"=w616:errorcluster)  [unwired: 7 in, 1 out]
      }
      frame "HeaterON" {
        n107 = Replace Array Subset(array=w623, new element=TRUE ("new element/subarray"), index=12) -> (w622:bool[])
        n108 = call-poly "Enqueue Message.vi"("error in (no error)"=w626, "Message"="Write bit pattern to FVIR and LDO", "Message Queue"=w630) -> ("error out"=w629:errorcluster)  [unwired: 7 in, 1 out]
      }
      frame "HeaterOFF" {
        n109 = Replace Array Subset(array=w636, new element=FALSE ("new element/subarray"), index=12) -> (w635:bool[])
        n110 = call-poly "Enqueue Message.vi"("error in (no error)"=w639, "Message"="Write bit pattern to FVIR and LDO", "Message Queue"=w643) -> ("error out"=w642:errorcluster)  [unwired: 7 in, 1 out]
      }
      frame "ResetFlowMeter_ON_LDO" {
        n111 = Replace Array Subset(array=w651, new element=TRUE ("new element/subarray"), index=13) -> (w650:bool[])
        n112 = call-poly "Enqueue Message.vi"("error in (no error)"=w647, "Message"="Write bit pattern to FVIR and LDO", "Message Queue"=w648) -> ("error out"=w646:errorcluster)  [unwired: 7 in, 1 out]
      }
      frame "ResetFlowMeter_OFF_LDO" {
        n113 = Replace Array Subset(array=w664, new element=FALSE ("new element/subarray"), index=13) -> (w663:bool[])
        n114 = call-poly "Enqueue Message.vi"("error in (no error)"=w660, "Message"="Write bit pattern to FVIR and LDO", "Message Queue"=w661) -> ("error out"=w659:errorcluster)  [unwired: 7 in, 1 out]
      }
      frame "Water_Heater_Status_ON_LDO" {
        n115 = Replace Array Subset(array=w677, new element=TRUE ("new element/subarray"), index=14) -> (w676:bool[])
        n116 = call-poly "Enqueue Message.vi"("error in (no error)"=w673, "Message"="Write bit pattern to FVIR and LDO", "Message Queue"=w674) -> ("error out"=w672:errorcluster)  [unwired: 7 in, 1 out]
      }
      frame "Water_Heater_Status_OFF_LDO" {
        n117 = Replace Array Subset(array=w690, new element=FALSE ("new element/subarray"), index=14) -> (w689:bool[])
        n118 = call-poly "Enqueue Message.vi"("error in (no error)"=w686, "Message"="Write bit pattern to FVIR and LDO", "Message Queue"=w687) -> ("error out"=w685:errorcluster)  [unwired: 7 in, 1 out]
      }
      frame "PID_Selector_ON" {
        n119 = Replace Array Subset(array=w703, new element=TRUE ("new element/subarray"), index=15) -> (w702:bool[])
        n120 = call-poly "Enqueue Message.vi"("error in (no error)"=w699, "Message"="Write bit pattern to FVIR and LDO", "Message Queue"=w700) -> ("error out"=w698:errorcluster)  [unwired: 7 in, 1 out]
      }
      frame "PID_Selector_OFF" {
        n121 = Replace Array Subset(array=w716, new element=FALSE ("new element/subarray"), index=15) -> (w715:bool[])
        n122 = call-poly "Enqueue Message.vi"("error in (no error)"=w712, "Message"="Write bit pattern to FVIR and LDO", "Message Queue"=w713) -> ("error out"=w711:errorcluster)  [unwired: 7 in, 1 out]
      }
      frame "MannequinGoToHomePos" {
        n123 = Replace Array Subset(array=w732, new element=TRUE ("new element/subarray"), index=9) -> (w731:bool[])
        n124 = call-poly "Enqueue Message.vi"("error in (no error)"=w734, "Message"="Write bit pattern to FVIR and LDO", "Message Queue"=w727) -> ("error out"=w729:errorcluster)  [unwired: 7 in, 1 out]
        n125 = call-poly "Enqueue Message.vi"("error in (no error)"=w729, "Message"="MannequinGoToHomePosClear", "Message Queue"=w727) -> ("error out"=w728:errorcluster)  [unwired: 7 in, 1 out]
      }
      frame "MannequinGoToHomePosClear" {
        n126 = Replace Array Subset(array=w743, new element=FALSE ("new element/subarray"), index=9) -> (w742:bool[])
        n127 = call-poly "Enqueue Message.vi"("error in (no error)"=w745, "Message"="Write bit pattern to FVIR and LDO", "Message Queue"=w749) -> ("error out"=w748:errorcluster)  [unwired: 7 in, 1 out]
      }
      frame "MannequinGoToWorkPos" {
        n128 = Replace Array Subset(array=w760, new element=TRUE ("new element/subarray"), index=10) -> (w759:bool[])
        n129 = call-poly "Enqueue Message.vi"("error in (no error)"=w762, "Message"="Write bit pattern to FVIR and LDO", "Message Queue"=w755) -> ("error out"=w757:errorcluster)  [unwired: 7 in, 1 out]
        n130 = call-poly "Enqueue Message.vi"("error in (no error)"=w757, "Message"="MannequinGoToWorkPosClear", "Message Queue"=w755) -> ("error out"=w756:errorcluster)  [unwired: 7 in, 1 out]
      }
      frame "MannequinGoToWorkPosClear" {
        n131 = Replace Array Subset(array=w771, new element=FALSE ("new element/subarray"), index=10) -> (w770:bool[])
        n132 = call-poly "Enqueue Message.vi"("error in (no error)"=w773, "Message"="Write bit pattern to FVIR and LDO", "Message Queue"=w777) -> ("error out"=w776:errorcluster)  [unwired: 7 in, 1 out]
      }
      frame "SpillCanGoToHomePos" {
        n133 = Replace Array Subset(array=w788, new element=TRUE ("new element/subarray"), index=11) -> (w787:bool[])
        n134 = call-poly "Enqueue Message.vi"("error in (no error)"=w790, "Message"="Write bit pattern to FVIR and LDO", "Message Queue"=w783) -> ("error out"=w785:errorcluster)  [unwired: 7 in, 1 out]
        n135 = call-poly "Enqueue Message.vi"("error in (no error)"=w785, "Message"="SpillCanGoToHomePosClear", "Message Queue"=w783) -> ("error out"=w784:errorcluster)  [unwired: 7 in, 1 out]
      }
      frame "SpillCanGoToHomePosClear" {
        n136 = Replace Array Subset(array=w799, new element=FALSE ("new element/subarray"), index=11) -> (w798:bool[])
        n137 = call-poly "Enqueue Message.vi"("error in (no error)"=w801, "Message"="Write bit pattern to FVIR and LDO", "Message Queue"=w805) -> ("error out"=w804:errorcluster)  [unwired: 7 in, 1 out]
      }
      frame "SpillCanGoToWorkPos" {
        n138 = Replace Array Subset(array=w816, new element=TRUE ("new element/subarray"), index=12) -> (w815:bool[])
        n139 = call-poly "Enqueue Message.vi"("error in (no error)"=w818, "Message"="Write bit pattern to FVIR and LDO", "Message Queue"=w811) -> ("error out"=w813:errorcluster)  [unwired: 7 in, 1 out]
        n140 = call-poly "Enqueue Message.vi"("error in (no error)"=w813, "Message"="SpillCanGoToWorkPosClear", "Message Queue"=w811) -> ("error out"=w812:errorcluster)  [unwired: 7 in, 1 out]
      }
      frame "SpillCanGoToWorkPosClear" {
        n141 = Replace Array Subset(array=w827, new element=FALSE ("new element/subarray"), index=12) -> (w826:bool[])
        n142 = call-poly "Enqueue Message.vi"("error in (no error)"=w829, "Message"="Write bit pattern to FVIR and LDO", "Message Queue"=w833) -> ("error out"=w832:errorcluster)  [unwired: 7 in, 1 out]
      }
      frame "TestCase1Winter" {
        # "Writing to PLC with value 1 at address 7"
        n143 = call-dynamic "Write Single Holding Register.vi"("error in"=w847, "register to write"=u16 1, "address"=u16 7 ("starting address"), "Modbus master in"=w845) -> ("error out"=w841:errorcluster, "Modbus master out"=w846:refnum<class "Modbus Master.lvclass">)  [unwired: 6 in]
        n144 = call-poly "Enqueue Message.vi"("error in (no error)"=w841, "Message"="Write bit pattern to FVIR and LDO", "Message Queue"=w842) -> ("error out"=w839:errorcluster)  [unwired: 7 in, 1 out]
      }
      frame "TestCase1Summer" {
        # "Writing to PLC with value 2 at address 7"
        n145 = call-dynamic "Write Single Holding Register.vi"("error in"=w861, "register to write"=u16 2, "address"=u16 7 ("starting address"), "Modbus master in"=w859) -> ("error out"=w855:errorcluster, "Modbus master out"=w860:refnum<class "Modbus Master.lvclass">)  [unwired: 6 in]
        n146 = call-poly "Enqueue Message.vi"("error in (no error)"=w855, "Message"="Write bit pattern to FVIR and LDO", "Message Queue"=w856) -> ("error out"=w853:errorcluster)  [unwired: 7 in, 1 out]
      }
      frame "TestCase2Winter" {
        # "Writing to PLC with value 3 at address 7"
        n147 = call-dynamic "Write Single Holding Register.vi"("error in"=w875, "register to write"=u16 3, "address"=u16 7 ("starting address"), "Modbus master in"=w873) -> ("error out"=w869:errorcluster, "Modbus master out"=w874:refnum<class "Modbus Master.lvclass">)  [unwired: 6 in]
        n148 = call-poly "Enqueue Message.vi"("error in (no error)"=w869, "Message"="Write bit pattern to FVIR and LDO", "Message Queue"=w870) -> ("error out"=w867:errorcluster)  [unwired: 7 in, 1 out]
      }
      frame "TestCase2Summer" {
        # "Writing to PLC with value 4 at address 7"
        n149 = call-dynamic "Write Single Holding Register.vi"("error in"=w889, "register to write"=u16 4, "address"=u16 7 ("starting address"), "Modbus master in"=w887) -> ("error out"=w883:errorcluster, "Modbus master out"=w888:refnum<class "Modbus Master.lvclass">)  [unwired: 6 in]
        n150 = call-poly "Enqueue Message.vi"("error in (no error)"=w883, "Message"="Write bit pattern to FVIR and LDO", "Message Queue"=w884) -> ("error out"=w881:errorcluster)  [unwired: 7 in, 1 out]
      }
      frame "TestCase3Winter" {
        # "Writing to PLC with value 5 at address 7"
        n151 = call-dynamic "Write Single Holding Register.vi"("error in"=w903, "register to write"=u16 5, "address"=u16 7 ("starting address"), "Modbus master in"=w901) -> ("error out"=w897:errorcluster, "Modbus master out"=w902:refnum<class "Modbus Master.lvclass">)  [unwired: 6 in]
        n152 = call-poly "Enqueue Message.vi"("error in (no error)"=w897, "Message"="Write bit pattern to FVIR and LDO", "Message Queue"=w898) -> ("error out"=w895:errorcluster)  [unwired: 7 in, 1 out]
      }
      frame "TestCase3Summer" {
        # "Writing to PLC with value 6 at address 7"
        n153 = call-dynamic "Write Single Holding Register.vi"("error in"=w917, "register to write"=u16 6, "address"=u16 7 ("starting address"), "Modbus master in"=w915) -> ("error out"=w911:errorcluster, "Modbus master out"=w916:refnum<class "Modbus Master.lvclass">)  [unwired: 6 in]
        n154 = call-poly "Enqueue Message.vi"("error in (no error)"=w911, "Message"="Write bit pattern to FVIR and LDO", "Message Queue"=w912) -> ("error out"=w909:errorcluster)  [unwired: 7 in, 1 out]
      }
      frame "TestCase4Winter" {
        # "Writing to PLC with value 7 at address 7"
        n155 = call-dynamic "Write Single Holding Register.vi"("error in"=w923, "register to write"=u16 7, "address"=u16 7 ("starting address"), "Modbus master in"=w930) -> ("error out"=w926:errorcluster, "Modbus master out"=w931:refnum<class "Modbus Master.lvclass">)  [unwired: 6 in]
        n156 = call-poly "Enqueue Message.vi"("error in (no error)"=w926, "Message"="Write bit pattern to FVIR and LDO", "Message Queue"=w927) -> ("error out"=w924:errorcluster)  [unwired: 7 in, 1 out]
      }
      frame "TestCase4Summer" {
        # "Writing to PLC with value 8 at address 7"
        n157 = call-dynamic "Write Single Holding Register.vi"("error in"=w945, "register to write"=u16 8, "address"=u16 7 ("starting address"), "Modbus master in"=w943) -> ("error out"=w939:errorcluster, "Modbus master out"=w944:refnum<class "Modbus Master.lvclass">)  [unwired: 6 in]
        n158 = call-poly "Enqueue Message.vi"("error in (no error)"=w939, "Message"="Write bit pattern to FVIR and LDO", "Message Queue"=w940) -> ("error out"=w937:errorcluster)  [unwired: 7 in, 1 out]
      }
      frame "ResetTestFVIR" {
        # "Writing to PLC with value 0 at address 7"
        n159 = call-dynamic "Write Single Holding Register.vi"("error in"=w959, "register to write"=u16 0, "address"=u16 7 ("starting address"), "Modbus master in"=w957) -> ("error out"=w953:errorcluster, "Modbus master out"=w958:refnum<class "Modbus Master.lvclass">)  [unwired: 6 in]
        n160 = call-poly "Enqueue Message.vi"("error in (no error)"=w953, "Message"="Write bit pattern to FVIR and LDO", "Message Queue"=w954) -> ("error out"=w951:errorcluster)  [unwired: 7 in, 1 out]
      }
      frame "ResetTestLDO" {
        # "Dont think this is used."
        # "Writing to PLC with value 0 at address 10"
        n161 = call-dynamic "Write Single Holding Register.vi"("error in"=w973, "register to write"=u16 0, "address"=u16 10 ("starting address"), "Modbus master in"=w971) -> ("error out"=w967:errorcluster, "Modbus master out"=w972:refnum<class "Modbus Master.lvclass">)  [unwired: 6 in]
        n162 = call-poly "Enqueue Message.vi"("error in (no error)"=w967, "Message"="Write bit pattern to FVIR and LDO", "Message Queue"=w968) -> ("error out"=w965:errorcluster)  [unwired: 7 in, 1 out]
      }
      frame "ConveyorON" {
        n163 = call-poly "Enqueue Message.vi"("error in (no error)"=w978, "Message"="Write bit pattern to FVIR and LDO", "Message Queue"=w977) -> ("error out"=w979:errorcluster)  [unwired: 7 in, 1 out]
        n164 = Replace Array Subset(array=w976, new element=TRUE ("new element/subarray"), index=0) -> (w975:bool[])
      }
      frame "ConveyorOFF" {
        n165 = call-poly "Enqueue Message.vi"("error in (no error)"=w990, "Message"="Write bit pattern to FVIR and LDO", "Message Queue"=w991) -> ("error out"=w992:errorcluster)  [unwired: 7 in, 1 out]
        n166 = Replace Array Subset(array=w988, new element=FALSE ("new element/subarray"), index=0) -> (w989:bool[])
      }
      frame "BlowerON" {
        n167 = call-poly "Enqueue Message.vi"("error in (no error)"=w1004, "Message"="Write bit pattern to FVIR and LDO", "Message Queue"=w1003) -> ("error out"=w1005:errorcluster)  [unwired: 7 in, 1 out]
        n168 = Replace Array Subset(array=w1002, new element=TRUE ("new element/subarray"), index=7) -> (w1001:bool[])
      }
      frame "BlowerOFF" {
        n169 = Replace Array Subset(array=w1015, new element=FALSE ("new element/subarray"), index=7) -> (w1014:bool[])
        n170 = call-poly "Enqueue Message.vi"("error in (no error)"=w1017, "Message"="Write bit pattern to FVIR and LDO", "Message Queue"=w1016) -> ("error out"=w1018:errorcluster)  [unwired: 7 in, 1 out]
      }
      frame "SendParamToPLCFVIR" {
        # "This for loop basically just takes the array from the Modbus queue and write\neach index value to each unique register. I.e. the first control value from the HMI\nwhich is \"Time delay of change direction of mannequin actuators\" is written to \nregister 1 (40002). The next control value from the HMI is the \"Number of\nmannequin movement\" and that value is written to register 2 (40003). \nThis continues until there are no further values in the array.\n\n(Register 0 is the bit combination from, regsiter 40001). See\nthe case  \"Writing to register 40001)"
        n171 = Variant To Data(type=i32[] [], Variant=w1039) -> (data=w1035:i32[], error out=w1032:errorcluster)  [unwired: 1 in]
        n172 = Array Size(array=w1035) -> (size(s)=w1036:i32)
        n173 = for {
          N: w1036 -> [_]
          tunnel: w1035 -> [w1050]
          shift-right: [w1044] -> w1033
          shift-left: w1034 -> [w1045]
          shift-right: [w1042] -> w1031
          shift-left: w1032 -> [w1043]
          i -> [w1048]
          n174 = Index Array(array=w1050, index=w1048) -> (element=w1049:i32)
          n175 = Add(x=1, y=w1048) -> (x+y=w1046:i32)
          n176 = call-dynamic "Write Single Holding Register.vi"("error in"=w1043, "register to write"=w1049, "address"=w1046, "Modbus master in"=w1045) -> ("error out"=w1042:errorcluster, "Modbus master out"=w1044:refnum<class "Modbus Master.lvclass">)  [unwired: 6 in]
        }
        n177 = call-poly "Enqueue Message.vi"("error in (no error)"=w1031, "Message"="Write bit pattern to FVIR and LDO", "Message Queue"=w1041) -> ("error out"=w1037:errorcluster)  [unwired: 7 in, 1 out]
      }
      frame "SendParamToPLCLDO" {
        # "This for loop basically just takes the array from the Modbus queue and write\neach index value to each unique register. I.e. the first control value from the HMI\nwhich is \"Time delay of change direction of mannequin actuators\" is written to \nregister 1 (40002). The next control value from the HMI is the \"Number of\nmannequin movement\" and that value is written to register 2 (40003). \nThis continues until there are no further values in the array.\n\n(Register 0 is the bit combination from, regsiter 40001). See\nthe case  \"Writing to register 40001)"
        n178 = Variant To Data(type=i32[] [], Variant=w1063) -> (data=w1060:i32[], error out=w1057:errorcluster)  [unwired: 1 in]
        n179 = call "Modbus Send Parameters LDO.vi"("error in (no error)"=w1057, "Array in"=w1060, "Modbus Master in"=w1059) -> ("error out"=w1056:errorcluster, "Modbus Master out"=w1058:refnum<class "Modbus Master.lvclass">)  [unwired: 7 in]
        n180 = call-poly "Enqueue Message.vi"("error in (no error)"=w1056, "Message"="Write bit pattern to FVIR and LDO", "Message Queue"=w1065) -> ("error out"=w1061:errorcluster)  [unwired: 7 in, 1 out]
      }
      frame "Reset all button signals to PLC" {
        # "Reset all the buttons signals after watchdog pause."
        n181 = call-dynamic "Write Multiple Holding Registers.vi"("error in"=w1076, "registers to write"=u16[] [99, 99, 99, 99, 99, 99, 99, 99, 99, 99, 99, 99], "starting address"=u16 10, "Modbus master in"=w1074) -> ("error out"=w1072:errorcluster, "Modbus master out"=w1075:refnum<class "Modbus Master.lvclass">)  [unwired: 6 in]
      }
      frame "Disconnect" {
        # "I moved this to the Exit State. Would like to eliminate the \"Connect\" and \"Disconnect\" button"
        # "Flushing the WD helper loop in order to quick close down, if the operator is pressing Exit"
        n182 = call-dynamic "Shutdown.vi"("error in"=w1088, "Modbus master in"=w1087) -> ("error out"=w1089:errorcluster)  [unwired: 9 in]
        n183 = call <vilib>:"Clear Errors.vi"("error in (no error)"=w1089) -> ("error out"=w1086:errorcluster)  [unwired: 5 in, 1 out]
        n184 = Flush Queue(queue=w1085, error in (no error)=w1086) -> (error out=w1082:errorcluster)  [unwired: 2 out]
        n185 = case shown="No Error" w1082 {
          selector: w1082 -> [w1098 w1101]
          tunnel: w1080 -> [w1090 w1099]
          tunnel: [w1096 w1100] -> w1081
          frame No Error {
            n186 = call-poly "Enqueue Message.vi"("error in (no error)"=w1098, "Message Data"="Succesfully disconnected with Modbus TCP/IP..." ("Acquiring and Logging..."), "Message"="Update Status - FVIR", "Message Queue"=w1090) -> ("error out"=w1097:errorcluster, "dup Message Queue"=w1095:refnum<queue>)  [unwired: 6 in]
            n187 = call-poly "Enqueue Message.vi"("error in (no error)"=w1097, "Message Data"="Succesfully disconnected with Modbus TCP/IP..." ("Acquiring and Logging..."), "Message"="Update Status - LDO", "Message Queue"=w1095) -> ("error out"=w1096:errorcluster)  [unwired: 6 in, 1 out]
          }
          frame Error {
            n188 = call-poly "Enqueue Message.vi"("error in (no error)"=w1101, "Message Data"="Error with disconnecting with Modbus TCP/IP..." ("Acquiring and Logging..."), "Message"="Update Status - FVIR", "Message Queue"=w1099) -> ("error out"=w1107:errorcluster, "dup Message Queue"=w1106:refnum<queue>)  [unwired: 6 in]
            n189 = call-poly "Enqueue Message.vi"("error in (no error)"=w1107, "Message Data"="Error with disconnecting with Modbus TCP/IP..." ("Acquiring and Logging..."), "Message"="Update Status - LDO", "Message Queue"=w1106) -> ("error out"=w1100:errorcluster)  [unwired: 6 in, 1 out]
          }
        }
      }
      frame "Exit" {
        # "Flushing the WD helper loop in order to quick close down, if the operator is pressing Exit"
        # "When main loop receive \"Exit\" on its queue, the exit case will commit \"Exit\" to its helper loop"
        # "Stop the VI"
        n190 = Flush Queue(queue=w1116, error in (no error)=w1117) -> (queue out=w1115:refnum<queue>, error out=w1114:errorcluster)  [unwired: 1 out]
        n191 = call-dynamic "Shutdown.vi"("error in"=w1114, "Modbus master in"=w1113) -> ("error out"=w1118:errorcluster)  [unwired: 9 in]
        n192 = call <vilib>:"Clear Errors.vi"("error in (no error)"=w1118) -> ("error out"=w1112:errorcluster)  [unwired: 5 in, 1 out]
        n193 = case shown="No Error" w1112 {
          selector: w1112 -> [w1136 w1139]
          tunnel: w1109 -> [w1128 w1137]
          tunnel: [w1134 w1138] -> w1111
          frame No Error {
            n194 = call-poly "Enqueue Message.vi"("error in (no error)"=w1136, "Message Data"="Succesfully disconnected with Modbus TCP/IP..." ("Acquiring and Logging..."), "Message"="Update Status - FVIR", "Message Queue"=w1128) -> ("error out"=w1135:errorcluster, "dup Message Queue"=w1133:refnum<queue>)  [unwired: 6 in]
            n195 = call-poly "Enqueue Message.vi"("error in (no error)"=w1135, "Message Data"="Succesfully disconnected with Modbus TCP/IP..." ("Acquiring and Logging..."), "Message"="Update Status - LDO", "Message Queue"=w1133) -> ("error out"=w1134:errorcluster)  [unwired: 6 in, 1 out]
          }
          frame Error {
            n196 = call-poly "Enqueue Message.vi"("error in (no error)"=w1139, "Message Data"="Error with disconnecting with Modbus TCP/IP..." ("Acquiring and Logging..."), "Message"="Update Status - FVIR", "Message Queue"=w1137) -> ("error out"=w1145:errorcluster, "dup Message Queue"=w1144:refnum<queue>)  [unwired: 6 in]
            n197 = call-poly "Enqueue Message.vi"("error in (no error)"=w1145, "Message Data"="Error with disconnecting with Modbus TCP/IP..." ("Acquiring and Logging..."), "Message"="Update Status - LDO", "Message Queue"=w1144) -> ("error out"=w1138:errorcluster)  [unwired: 6 in, 1 out]
          }
        }
        n198 = call-poly "Enqueue Message.vi"("Priority Message? (F)"=TRUE, "error in (no error)"=w1111, "Message"="Exit", "Message Queue"=w1115) -> ("error out"=w1123:errorcluster)  [unwired: 6 in, 1 out]
        n199 = Release Queue(queue=w1127, error in (no error)=w1123) -> (error out=w1110:errorcluster)  [unwired: 1 in, 2 out]
      }
      frame "ValveChangeEPV" {
        n200 = Variant To Data(error in=w1159, type=0.0 ("Numeric"), Variant=w1158) -> (data=w1156:dbl, error out=w1157:errorcluster)
        n201 = call "UTILITY Modbus 32bit Number to 16bit Array.vi"("error in"=w1157, "32-bit IEEE 754"=w1156) -> ("error out"=w1155:errorcluster, "U16 Array Representation"=w1153:u16[])  [unwired: 8 in]
        n202 = call-dynamic "Write Multiple Holding Registers.vi"("error in"=w1155, "registers to write"=w1153, "starting address"=u16 11 ("address"), "Modbus master in"=w1152) -> ("error out"=w1149:errorcluster, "Modbus master out"=w1151:refnum<class "Modbus Master.lvclass">)  [unwired: 6 in]
        n203 = call-poly "Enqueue Message.vi"("error in (no error)"=w1149, "Message"="Write bit pattern to FVIR and LDO", "Message Queue"=w1147) -> ("error out"=w1148:errorcluster)  [unwired: 7 in, 1 out]
      }
      frame "TempChangeDRK375" {
        n204 = Variant To Data(error in=w1178, type=0.0 ("Numeric"), Variant=w1177) -> (data=w1172:dbl, error out=w1173:errorcluster)
        n205 = call "UTILITY Modbus 32bit Number to 16bit Array.vi"("error in"=w1173, "32-bit IEEE 754"=w1172) -> ("error out"=w1176:errorcluster, "U16 Array Representation"=w1174:u16[])  [unwired: 8 in]
        n206 = call-dynamic "Write Multiple Holding Registers.vi"("error in"=w1176, "registers to write"=w1174, "starting address"=u16 13 ("address"), "Modbus master in"=w1171) -> ("error out"=w1167:errorcluster, "Modbus master out"=w1170:refnum<class "Modbus Master.lvclass">)  [unwired: 6 in]
        n207 = call-poly "Enqueue Message.vi"("error in (no error)"=w1167, "Message"="Write bit pattern to FVIR and LDO", "Message Queue"=w1168) -> ("error out"=w1166:errorcluster)  [unwired: 7 in, 1 out]
      }
      frame "ValveChangeDRK375" {
        n208 = Variant To Data(error in=w1197, type=0.0 ("Numeric"), Variant=w1196) -> (data=w1191:dbl, error out=w1192:errorcluster)
        n209 = call "UTILITY Modbus 32bit Number to 16bit Array.vi"("error in"=w1192, "32-bit IEEE 754"=w1191) -> ("error out"=w1195:errorcluster, "U16 Array Representation"=w1194:u16[])  [unwired: 8 in]
        n210 = call-dynamic "Write Multiple Holding Registers.vi"("error in"=w1195, "registers to write"=w1194, "starting address"=u16 15 ("address"), "Modbus master in"=w1190) -> ("error out"=w1186:errorcluster, "Modbus master out"=w1189:refnum<class "Modbus Master.lvclass">)  [unwired: 6 in]
        n211 = call-poly "Enqueue Message.vi"("error in (no error)"=w1186, "Message"="Write bit pattern to FVIR and LDO", "Message Queue"=w1187) -> ("error out"=w1185:errorcluster)  [unwired: 7 in, 1 out]
      }
      frame "Output_Temperature_Target" {
        n212 = Variant To Data(error in=w1211, type=0.0 ("Numeric"), Variant=w1210) -> (data=w1214:dbl, error out=w1215:errorcluster)
        n213 = call "UTILITY Modbus 32bit Number to 16bit Array.vi"("error in"=w1215, "32-bit IEEE 754"=w1214) -> ("error out"=w1217:errorcluster, "U16 Array Representation"=w1216:u16[])  [unwired: 8 in]
        n214 = call-dynamic "Write Multiple Holding Registers.vi"("error in"=w1217, "registers to write"=w1216, "starting address"=u16 17 ("address"), "Modbus master in"=w1209) -> ("error out"=w1206:errorcluster, "Modbus master out"=w1208:refnum<class "Modbus Master.lvclass">)  [unwired: 6 in]
        n215 = call-poly "Enqueue Message.vi"("error in (no error)"=w1206, "Message"="Write bit pattern to FVIR and LDO", "Message Queue"=w1204) -> ("error out"=w1205:errorcluster)  [unwired: 7 in, 1 out]
      }
      frame "Output_Flow_Target" {
        n216 = Variant To Data(error in=w1230, type=0.0 ("Numeric"), Variant=w1229) -> (data=w1233:dbl, error out=w1234:errorcluster)
        n217 = call "UTILITY Modbus 32bit Number to 16bit Array.vi"("error in"=w1234, "32-bit IEEE 754"=w1233) -> ("error out"=w1236:errorcluster, "U16 Array Representation"=w1235:u16[])  [unwired: 8 in]
        n218 = call-dynamic "Write Multiple Holding Registers.vi"("error in"=w1236, "registers to write"=w1235, "starting address"=u16 31 ("address"), "Modbus master in"=w1228) -> ("error out"=w1225:errorcluster, "Modbus master out"=w1227:refnum<class "Modbus Master.lvclass">)  [unwired: 6 in]
        n219 = call-poly "Enqueue Message.vi"("error in (no error)"=w1225, "Message"="Write bit pattern to FVIR and LDO", "Message Queue"=w1223) -> ("error out"=w1224:errorcluster)  [unwired: 7 in, 1 out]
      }
    }
    n220 = case shown="False" "Read States" {
      tunnel: w12 -> [w38 w41]
      tunnel: w11 -> [_ w40]
      tunnel: [w38 w39] -> w10
      frame False {
      }
      frame True {
        n221 = Build Array (concatenate)(w41, w40) -> (w39:string[])
        "States" <- w39
      }
    }
    n222 = call "Error Handler - Message Handling Loop.vi"("error in (no error)"=w22, "Message Queue"=w30) -> ("dup error in"=w34:errorcluster)  [unwired: 8 in, 1 out]
    "Loop Count" <- w13
  }
  n223 = Merge Errors(w3) -> (→"error out":errorcluster)
